vi "WHD_VEten_0.2.vi"() -> ()   [LabVIEW 2015]
uses:
  <vilib>/RTwatchdog.llb/Watchdog expiration actions.ctl
  <vilib>/LabVIEW Targets/FPGA/cRIO/shared/nicrio_ModuleControls/nicrio_cRIO-9234_DataRatesRing2.ctl
  <vilib>/userdefined/High Color/nirio_resource_hc.ctl
  <vilib>/FPGAPlugInAG/cRIO-9031/niLvFpga_Open_cRIO-9031.vi
  <vilib>/Utility/file.llb/Write Delimited Spreadsheet (string).vi
  <vilib>/real-time/rtutility.llb/RT Restart Target (Self).vi
  <vilib>/FPGAPlugInAG/cRIO-9031/niLvFpga_Run_cRIO-9031.vi
  <vilib>/Utility/error.llb/Error Cluster From Error Code.vi
  <vilib>/rvi/errors/niLvFpgaAdjustHostInterfaceError.vi
  <vilib>/rvi/interface/common/niFpgaWaitOnOcc.vi
  <vilib>/FPGAPlugInAG/cRIO-9031/niLvFpga_Reset_cRIO-9031.vi
  <vilib>/Utility/file.llb/Read Delimited Spreadsheet (string).vi
  <vilib>/FPGAPlugInAG/cRIO-9031/niLvFpga_Close_cRIO-9031.vi
  <vilib>/rvi/interface/nirviOpenFPGA/nirviOpenFPGA.xnode
  FPGA Bitfiles/W&RDEuskotrenIBA_FPGATarget2_FPGA8aws_YNPuKjtl2tk.lvbitx
  <vilib>/rvi/interface/nirviMethod/nirviMethod.xnode
  <vilib>/rvi/interface/nirviReadWriteControl/nirviReadWriteControl.xnode
  <vilib>/rvi/interface/nirviCloseFPGA/nirviCloseFPGA.xnode
  <vilib>/real-time/NI_Real-Time Libraries.lvlib
  <vilib>/NI_Real-Time Target Support.lvlib
  NiFpgaLv.dll
  <vilib>/rvi/errors/niLvFpgaMergeErrorWithErrorCode.vi
  AURA_Wheel/Json2Labv.lvlib
  AURA_Wheel/AuraWheelAPI/AuraWheel.lvlib
  <vilib>/FPGAPlugInAG/cRIO-9031/niLvFpga_ConfigureFifo_cRIO-9031.vi
  <vilib>/FPGAPlugInAG/cRIO-9031/niLvFpga_StartFifo_cRIO-9031.vi
  <vilib>/FPGAPlugInAG/cRIO-9031/niLvFpga_ReadFifo_cRIO-9031.vi
  <vilib>/FPGAPlugInAG/cRIO-9031/niLvFpga_StopFifo_cRIO-9031.vi
panel:
  out "error out":errorcluster
  in  "TIEMPO SUBIDA FALLOS (MS)":u16=13
  out "all rows":string[][](array[string])
  out "Response headers 2":string
  in  "Parametros AuraWheel 2":string[](array[string])=["JOH653JDBHGGA4111LOMJG", "WRD03NEM", "http://api.aurawheel.sb/services/wrd/upload"]
  out "data 2":cluster{"status":string}
  out "JSON String Out 2":string
  in  "DC CONTROL":bool
  out "JSON String Out":string
  out "WHEEL_SENSOR":bool=TRUE
  out "Series del convoy":string[](array[string])
  out "it-read-LR6":i32[](array[numeric])
  out "it-LR6":i32
  out "Ejes_convoy":i32
  out "Nº Ejes":i32[](array[numeric])
  out "Plataformas?":bool
  out "TAGs LR6":string[](array[string])
  out "Series_flota":string[](array[string])
  out "Tabla_flota":string[][](array[string])
  out "Puntos medios de las ventanas":dbl[][](array[numeric])
  out "configuration file path":path=path "c:/Parametros.cfg"
  in  "IP synchr":string
  in  "Canal ccero?":bool
  in  "Digital?":bool=TRUE
  out "Numeric 3":i32
  out "TAGs HEX":string[](array[string])
  out "data":cluster{"status":string}
  out "confRFID":path=path "c:/RFID/TAGS.csv"
  out "TAGS leidos":path=path "c:/RFID/TAGS.csv"
  in  "Use Aura?":bool
  in  "Parametros AuraWheel":string[](array[string])
  in  "Parámetros acelerómetros":dbl[](array[numeric])
  out "RFID_Error 2":errorcluster
  out "Acelerómetros OK?":bool[](array[boolean])
  out "Fin":bool
  out "Contador":i32=1
  in  "expiration actions":T1={"reset"=TRUE, "occurrence"=FALSE, "trigger protocol"=enum."active high", "trigger line"=enum."none", "disable watchdog on VI exit"=FALSE}
  out "Path TEST":path=path "c:/TEST"
  out "Fallo fotocelula":bool
  out "Path_Borrar":path=path "c:/Trenes"
  out "Longitud de la unidad":dbl
  out "Bucle Espera":i32
  out "Aviso no detección":string
  out "Time to Acquire Block (ms)":i32
  out "Distancia de acelerómetros":dbl[](array[numeric])
  out "Block Size":u32
  out "Distancias generales":dbl[](array[numeric])
  in  "Reset del controlador":bool
  in  "Configuración":bool
  in  "Parar la aplicación":bool
  out "Acel 4":bool=TRUE
  out "Acel 3":bool=TRUE
  out "Acel 2":bool=TRUE
  out "Acel 1":bool=TRUE
  out "RFID":bool=TRUE
  out "date/time string":string
  out "Obstruido?":bool
  out "Tiempo":dbl
  out "Inicio pasada":timestamp
  out "Ultimo TEST":timestamp
  out "Fuente":bool=TRUE
  out "Estado":string
  in  "Number of Channels":u32=9
  out "RFID_ID":refnum<k5>
  out "DC OK":string
  out "Aviso temperatura":string
  in  "Tab Control":T2(tab)=enum."Parámetros"
  out "UT":dbl
  out "V (m/s)":dbl
  out "Temperatura (ºC)":dbl
  out "Max RMS Ruedas":dbl[][](array[numeric])
  in  "Hora de borrado":string
  out "result":bool
  out "TAGs":string[](array[string])
  out "TAGs_AURAwheel":string[][](array[string])
  out "Nombre de archivo":path[](array[path])
  out "Tiempo de paso (s)":dbl
  out "Tiempo extra de adquisición (s)":dbl
  out "Número de ejes detectados":i32
  out "Buffer Underflow":bool
  out "Buffer Overflow":bool
  out "Disco Duro Disponible (bytes)":i64
  out "Path Pasada":path
  out "Fallo sensores":string
  out "T fuera rango":bool
  in  "Frecuencia de muestreo (Hz)":dbl=25600.0
  in  "Escaneos de la FIFO por canal":u32=4000
  in  "Tiempo extra al detector de paso (s)":dbl=1.0
  in  "Filtro digital (ms)":u16=13
  in  "dt RMS":dbl=256.0
  in  "Frecuencia de muestreo y módulo CRIO":T3=2 items=["51.200 kS/s (NI 9234)"=1, "25.600 kS/s (NI 9234)"=2, "17.067 kS/s (NI 9234)"=3, "12.800 kS/s (NI 9234)"=4, "10.240 kS/s (NI 9234)"=5, "8.533 kS/s (NI 9234)"=6, "7.314 kS/s (NI 9234)"=7, "6.400 kS/s (NI 9234)"=8, "5.689 kS/s (NI 9234)"=9, "5.120 kS/s (NI 9234)"=10, "4.654 kS/s (NI 9234)"=11, "4.267 kS/s (NI 9234)"=12, "3.938 kS/s (NI 9234)"=13, "3.657 kS/s (NI 9234)"=14, "3.413 kS/s (NI 9234)"=15, "3.200 kS/s (NI 9234)"=16, "3.012 kS/s (NI 9234)"=17, "2.845 kS/s (NI 9234)"=18, "2.695 kS/s (NI 9234)"=19, "2.560 kS/s (NI 9234)"=20, "2.438 kS/s (NI 9234)"=21, "2.328 kS/s (NI 9234)"=22, "2.226 kS/s (NI 9234)"=23, "2.133 kS/s (NI 9234)"=24, "2.048 kS/s (NI 9234)"=25, "1.969 kS/s (NI 9234)"=26, "1.896 kS/s (NI 9234)"=27, "1.829 kS/s (NI 9234)"=28, "1.765 kS/s (NI 9234)"=29, "1.707 kS/s (NI 9234)"=30, "1.652 kS/s (NI 9234)"=31]
  in  "Puerto RFID":u16=2189
  in  "IP RFID":string="192.168.106.99"
  in  "Offset_rueda":fxp<+/-,24,-4>=0.004999998956918716 format="%.27g"
  in  "Count(mSec)":u32=2
  in  "LR6 IP address":string="192.168.106.94"
  in  "Port LR6":u16=2001
  in  "LIMITE MAX":dbl
  in  "LIMITE MIN":dbl
  in  "TIMEOUT":u16=2189
  in  "BYTES TO READ":u16=2189
  in  "DEVICE ADDRESS":u16=2189
  in  "Nº ACELEROMETROS":u16=13
  in  "Nº INDUCTIVOS":u16=13
  in  "Nº MAX ARCHIVOS":u16=13
  in  "MB MIN MEMORIA LIBRE":dbl=13.0 format="%#_10g"
  in  "MB LIBRE OK":dbl=13.0 format="%#_10g"
  in  "RFID_NEM_On":bool
  in  "RFID_GEN_On":bool
  in  "WDOG RESET":bool
  in  "WDOG DISABLE":bool
  out "ID DISPOSITIVO":string
  in  "HORA_SUBIDA_FALLOS":string="08:51 AM"
  out "time string 3":string
  in  "HORA_FINAL_SUBIDA":string="08:51 AM"
  in  "Pruebas RFID 2":bool
  in  "Pruebas RFID 1":bool
  in  "Descargar":bool
  out "Parámetros":bool=TRUE
  out "Distacias y medidas de dispositivos":bool=TRUE
  out "RFID_Error":errorcluster
  out "error FPGA":errorcluster
  out "error manipulacion archivos":errorcluster
  out "Unidades y ejes":bool=TRUE
  out "RFID":bool=TRUE
  out "error AURA":errorcluster
  out "Response headers":string
  out "RFID_LR6_Error":errorcluster
  # "Funciona?"
  # "Inductivo"
  # "A4"
  # "A3"
  # "A1"
  # "A2"
  # "Última detección de unidad"
  # "Error!!"
  # "Estado de la memoria"
  # "Espera"
  # "Adquisicion"
  # "Adquisicion"
  # "Procesado"
  # "Procesado"
  # "Procesado"
  # "Procesado"
  # "Procesado"
  # "Parámetros de configuración"
  # "Límites Acelerómetros"
  # "Parámetros de muestreo"
  # "Parámetros de adquisición"
  # "Parámetros de procesado"
  # "Descarga de planos y TEST"
  # "NO"
  # "SI"
  # "Descarga archivos binarios de adquisición"
  # "NO"
  # "SI"
  # "Cargar datos de configuración"
  # "Errores!!"
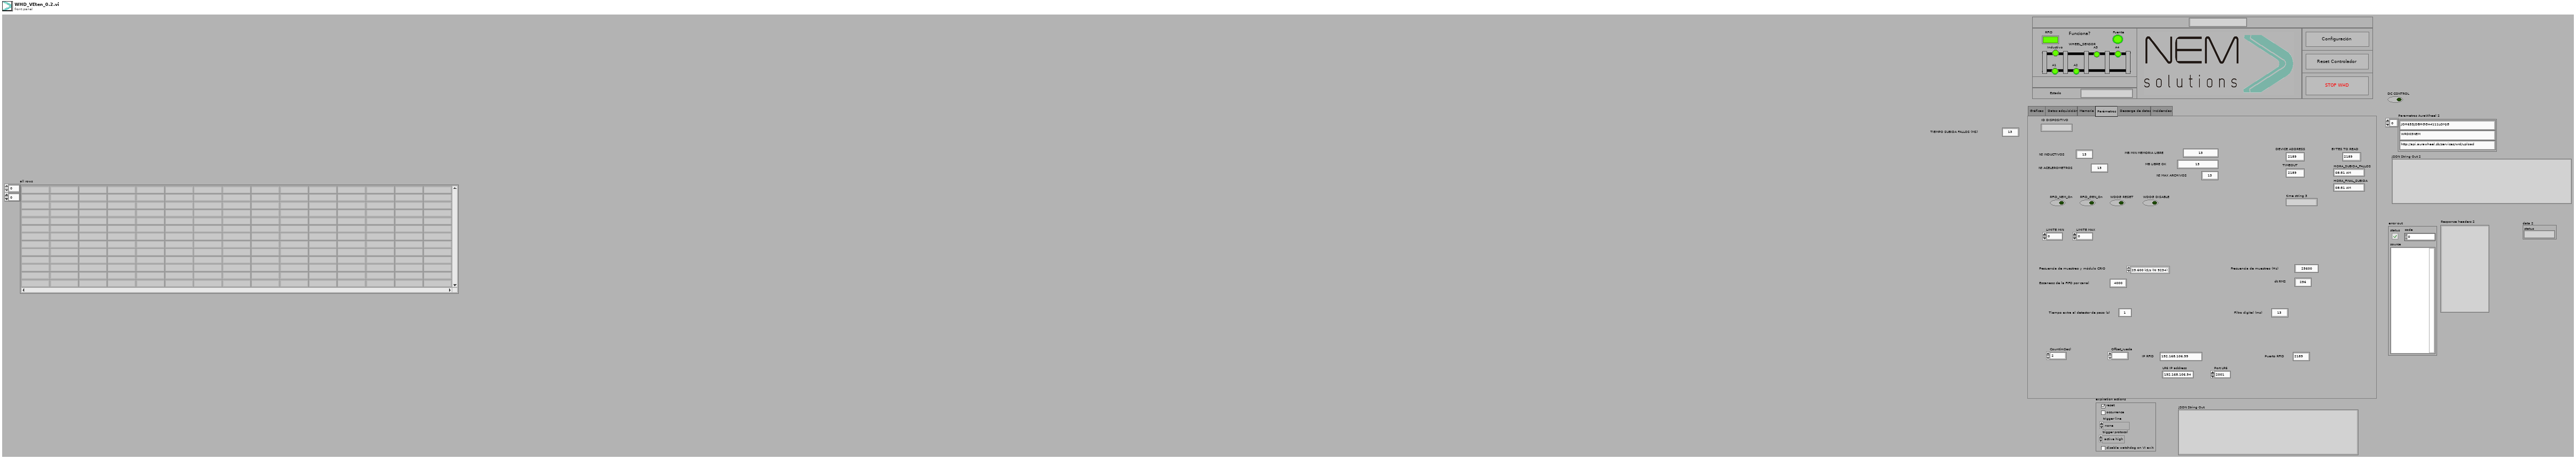
[diagram p1: front panel]
types:
  T1 = typedef "Watchdog expiration actions.ctl" = cluster{"reset":bool, "occurrence":bool, "trigger protocol":enum16{"active high", "active low", "open collector"}, "trigger line":enum16{"none", "line 0", "line 1", "line 2", "line 3", "line 4", "line 5", "line 6", "line 7", "SMB line 0"}, "disable watchdog on VI exit":bool}
  T2 = enum32{"Gráficas", "Datos adquisición", "Memoria", "Parámetros", "Descarga de datos", "Incidencias"}
  T3 = typedef "nicrio_cRIO-9234_DataRatesRing2.ctl" = u8
  T4 = typedef "nirio_resource_hc.ctl" = tag
  T5 = enum16{"Standard", "Buffered", "CRLF", "Immediate"}
  T6 = enum16{"open", "replace", "create", "open or create", "replace or create", "replace or create with confirmation"}
  T7 = enum16{"big-endian, network order", "native, host order", "little-endian"}
  T8 = cluster{"error IO":errorcluster, bool[], u32[], string[], dbl[]}
  T9 = cluster{"g_ts":dbl, "p_sp":dbl, "p_tp":dbl, "p_tg":cluster{"tg_n":dbl, "tg_t":string}[], "p_ax":cluster{"ax_n":dbl, "ax_sp":dbl, "ax_wh":cluster{"wh_p":dbl, "wh_a1":dbl, "wh_a2":dbl, "wh_a3":dbl, "wh_a4":dbl}[]}[]}
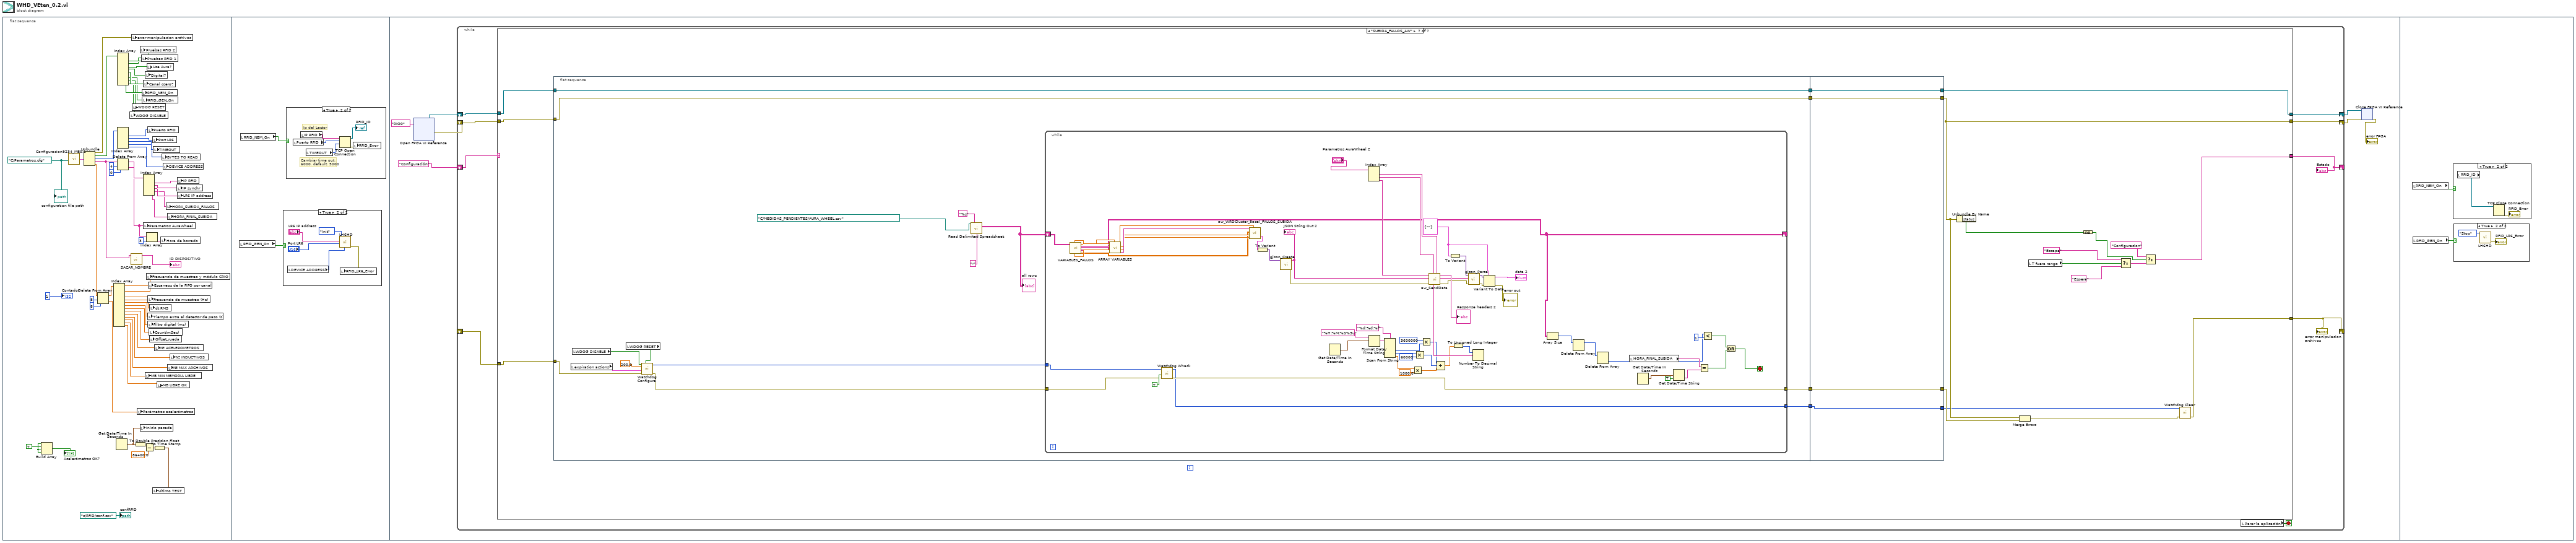
[diagram p0: block diagram]
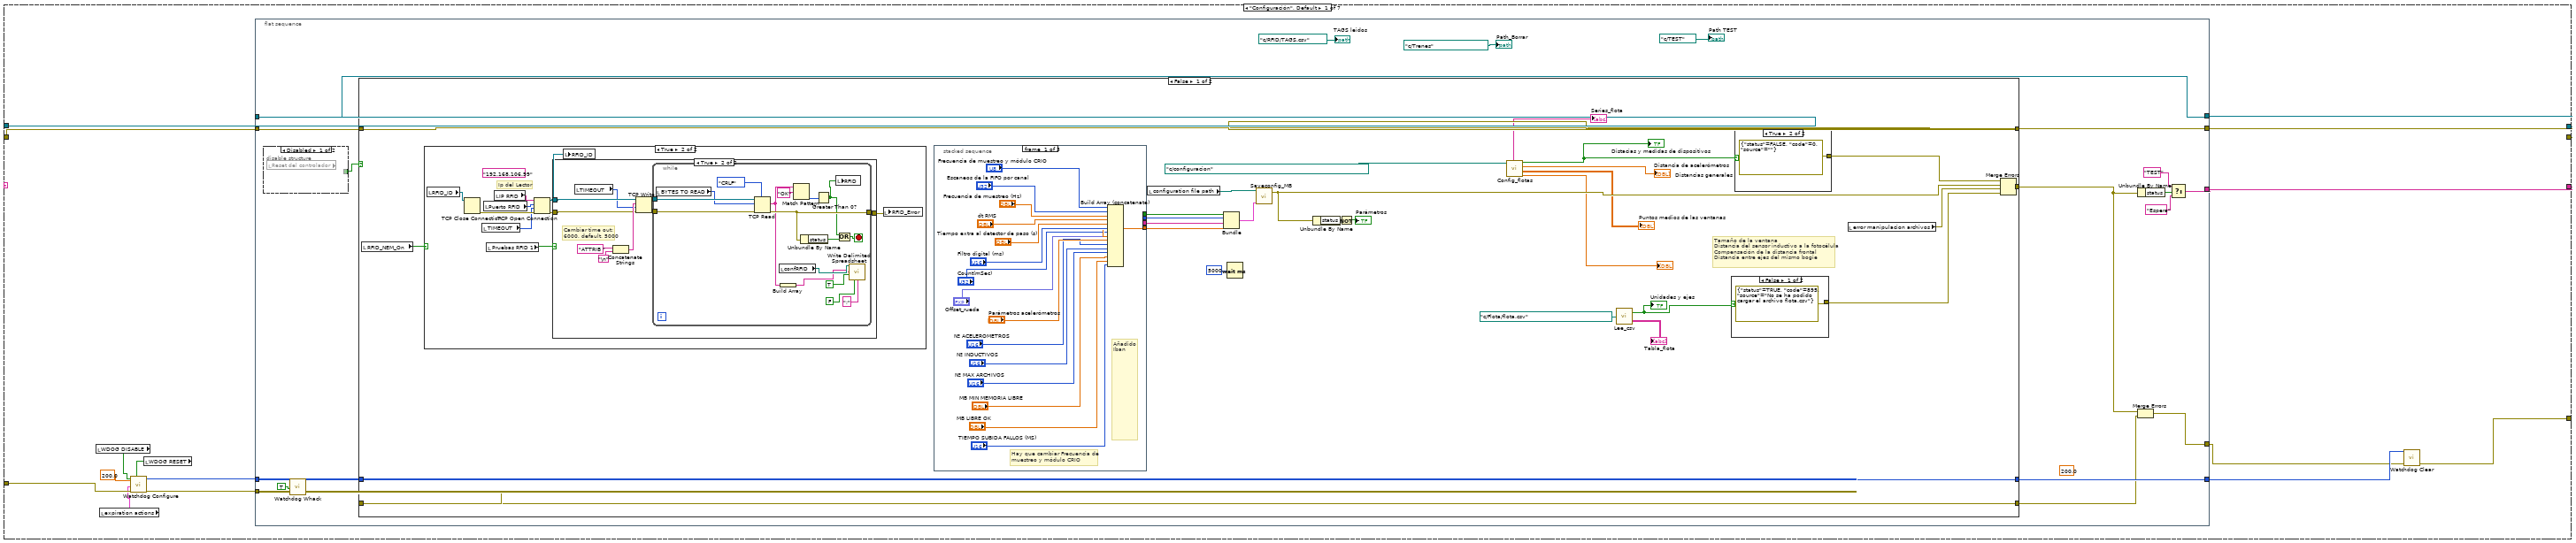
[diagram p4: hidden frame]
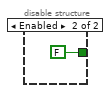
[diagram p5: hidden frame]
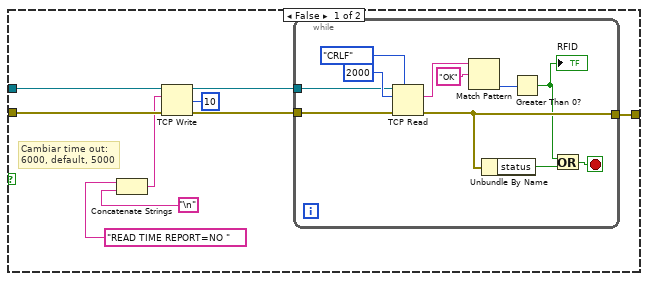
[diagram p7: hidden frame]
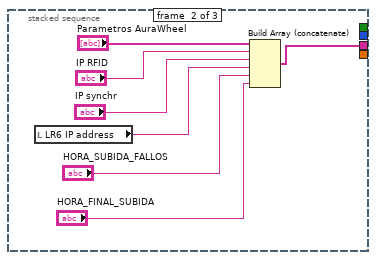
[diagram p8: hidden frame]
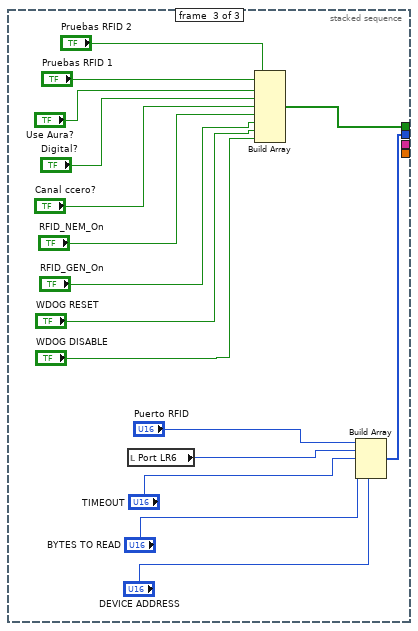
[diagram p9: hidden frame]
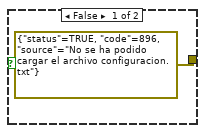
[diagram p10: hidden frame]
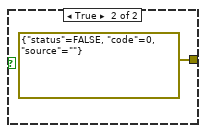
[diagram p11: hidden frame]
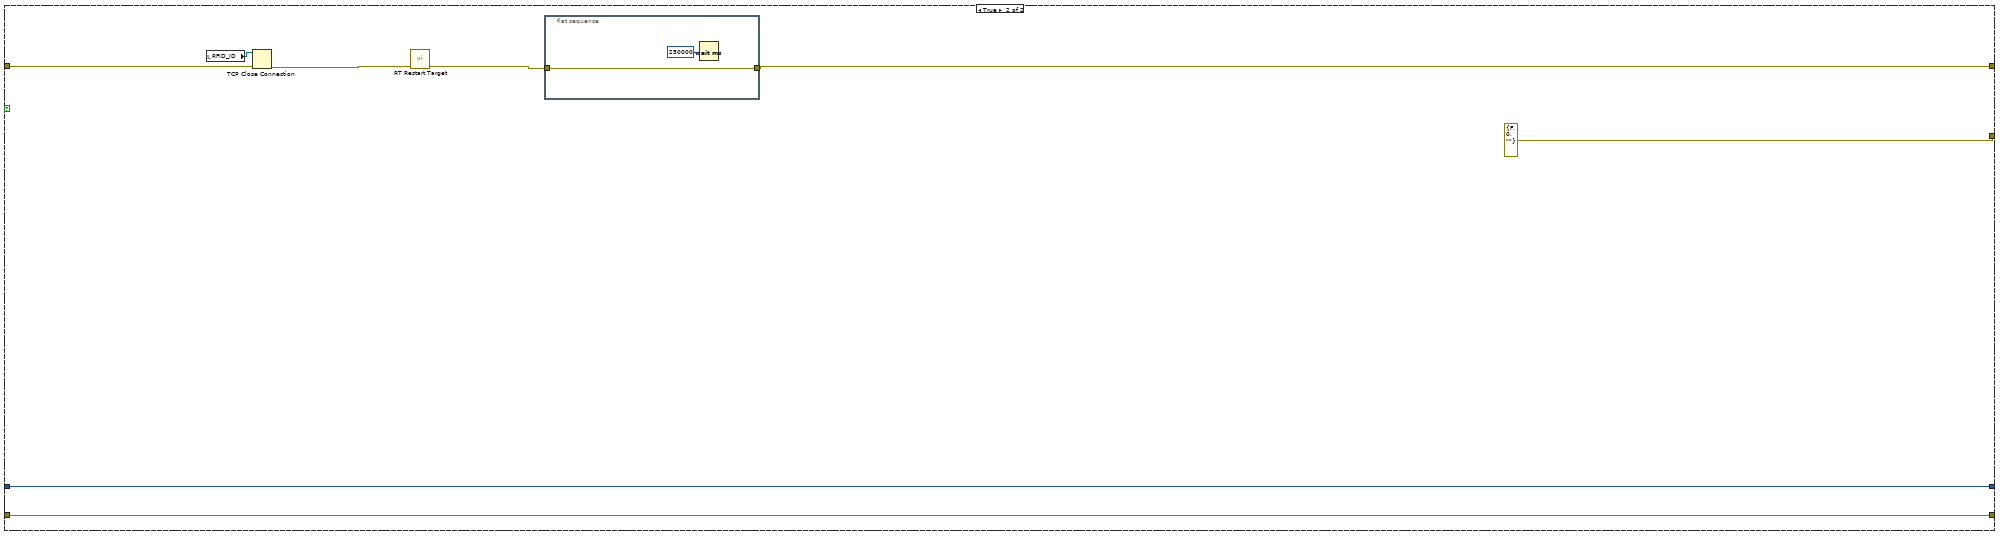
[diagram p12: hidden frame]
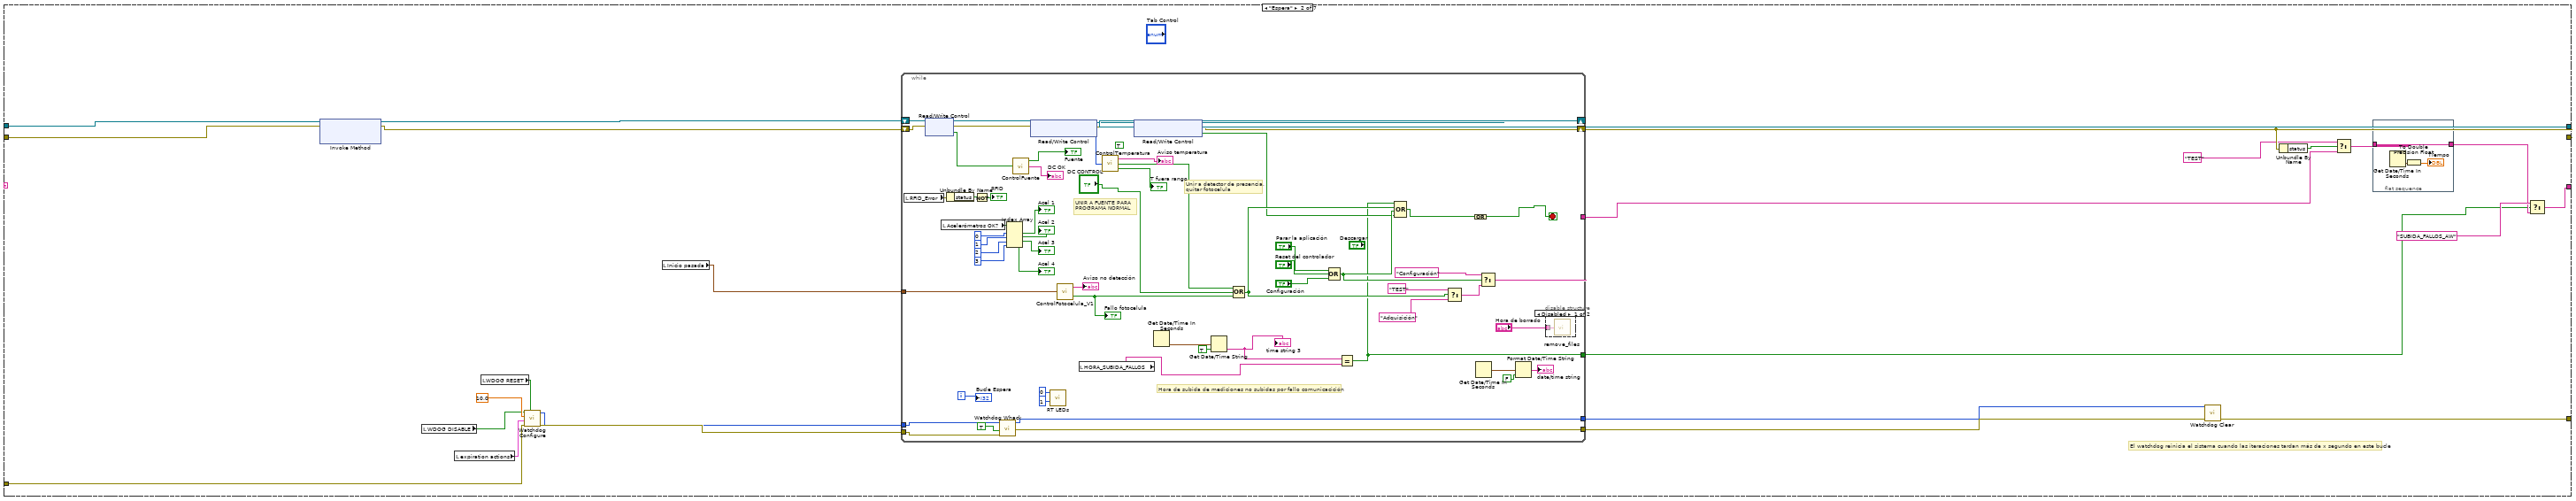
[diagram p13: hidden frame]
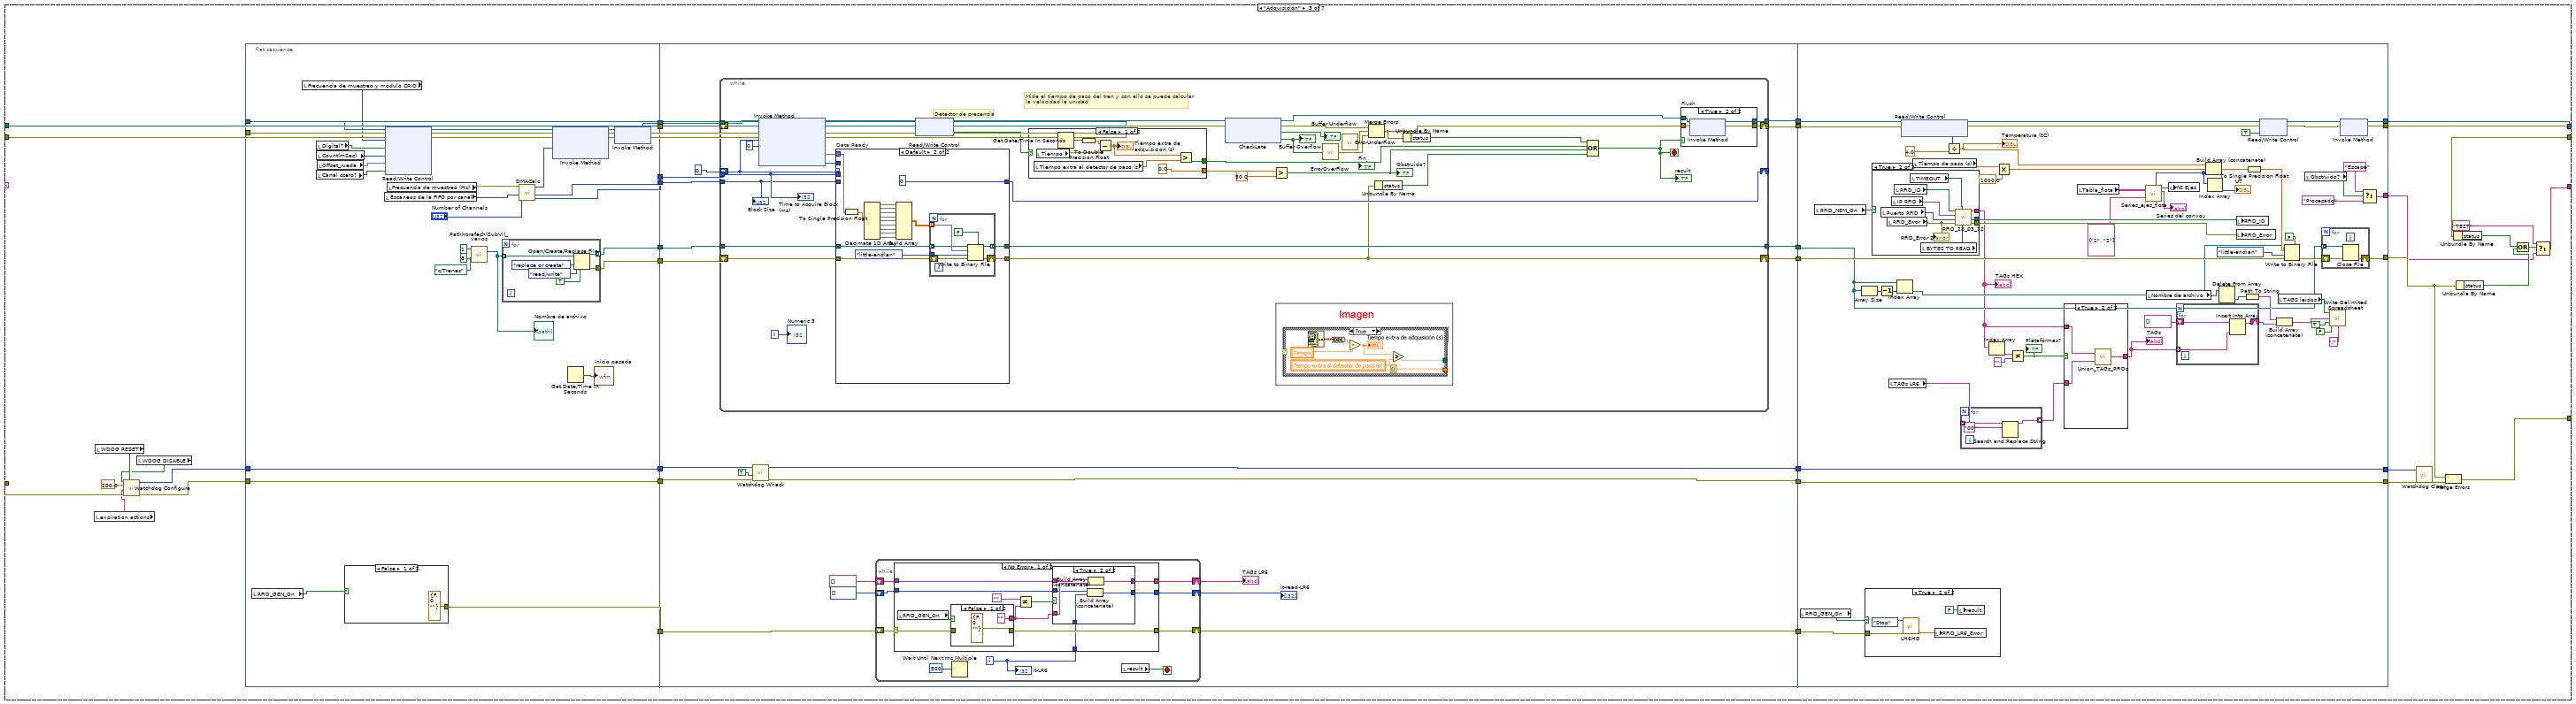
[diagram p15: hidden frame]
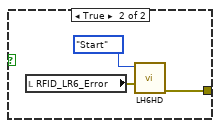
[diagram p16: hidden frame]
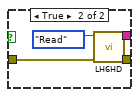
[diagram p17: hidden frame]
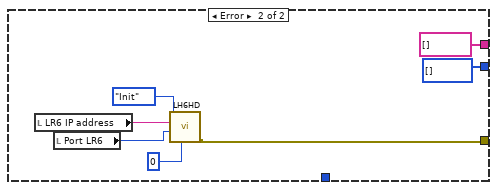
[diagram p19: hidden frame]
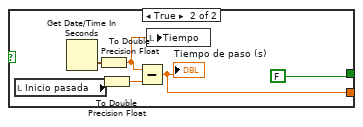
[diagram p20: hidden frame]
diagram:
  n1 = flat-sequence {
    frame #0 {
      w43 = TRUE
      w17 = path "C:/Parametros.cfg" ("configuration file path")
      n2 = Build Array(w43, w43, w43, w43) -> (→"Acelerómetros OK?":bool[])
      n3 = call "Configuracion9234_MB0.1.vi"("configuration file path"=w17) -> ("output cluster"=w40:T8)
      n4 = Unbundle(w40) -> ("error IO"=w46:errorcluster, w45:bool[], w44:u32[], w16:string[], w38:dbl[])
      n5 = Delete From Array(array=w38, length=8, index=8) -> (deleted portion=w34:dbl[], array with subset deleted=w37:dbl[])
      n6 = Index Array(array=w37) -> (element #1=w54:dbl, element #2=w53:dbl, element #3=w52:dbl, element #4=w51:dbl, element #5=w50:dbl, element #6=w49:dbl, element #7=w25:dbl, element #8=w24:dbl, element #9=w7:dbl, element #10=w6:dbl, element #11=w5:dbl, element #12=w4:dbl, element #13=w3:dbl)  [unwired: 13 in]
      n7 = Get Date/Time In Seconds() -> (seconds since 1Jan1904=w56:timestamp)
      n8 = Index Array(array=w45) -> (element #1=w48:bool, element #2=w47:bool, element #3=w33:bool, element #4=w21:bool, element #5=w26:bool, element #6=w11:bool, element #7=w10:bool, element #8=w9:bool, element #9=w8:bool)  [unwired: 9 in]
      n9 = Index Array(array=w44) -> (element #1=w39:u32, element #2=w18:u32, element #3=w14:u32, element #4=w13:u32, element #5=w12:u32)  [unwired: 5 in]
      n10 = Delete From Array(array=w16, length=4, index=0) -> (deleted portion=w22:string[], array with subset deleted=w32:string[])
      n11 = local write "WDOG DISABLE"(w8) -> ()
      n12 = call "SACAR_NOMBRE.vi"("Array 2"=w16) -> ("deleted portion"=→"ID DISPOSITIVO":string)  [unwired: 9 in]
      n13 = local write "error manipulacion archivos"(w46) -> ()
      n14 = local write "WDOG RESET"(w9) -> ()
      n15 = To Double Precision Float(number=w56) -> (double precision float=w58:dbl)
      n16 = local write "Parámetros acelerómetros"(w34) -> ()
      n17 = local write "Pruebas RFID 2"(w48) -> ()
      n18 = local write "Inicio pasada"(w56) -> ()
      n19 = local write "Pruebas RFID 1"(w47) -> ()
      n20 = local write "RFID_NEM_On"(w11) -> ()
      n21 = local write "RFID_GEN_On"(w10) -> ()
      n22 = local write "Canal ccero?"(w26) -> ()
      n23 = Index Array(array=w32) -> (element #1=w20:string, element #2=w23:string, element #3=w19:string, element #4=w2:string, element #5=w1:string)  [unwired: 5 in]
      n24 = local write "Parametros AuraWheel"(w22) -> ()
      n25 = Subtract(x=w58, y=86400.0) -> (x-y=w57:dbl)
      n26 = local write "Digital?"(w21) -> ()
      n27 = local write "MB MIN MEMORIA LIBRE"(w4) -> ()
      n28 = Index Array(array=w22, index=3) -> (element=w27:string)
      n29 = local write "Frecuencia de muestreo y módulo CRIO"(w54) -> ()
      n30 = local write "Use Aura?"(w33) -> ()
      n31 = local write "Tiempo extra al detector de paso (s)"(w50) -> ()
      n32 = local write "Puerto RFID"(w39) -> ()
      n33 = local write "Frecuencia de muestreo (Hz)"(w52) -> ()
      n34 = local write "Filtro digital (ms)"(w49) -> ()
      n35 = local write "Escaneos de la FIFO por canal"(w53) -> ()
      n36 = local write "Count(mSec)"(w25) -> ()
      n37 = local write "dt RMS"(w51) -> ()
      n38 = local write "Offset_rueda"(w24) -> ()
      n39 = local write "Port LR6"(w18) -> ()
      n40 = local write "TIMEOUT"(w14) -> ()
      n41 = To Time Stamp(1:w57) -> (0:w55:timestamp)
      n42 = local write "Ultimo TEST"(w55) -> ()
      n43 = local write "Nº ACELEROMETROS"(w7) -> ()
      n44 = local write "MB LIBRE OK"(w3) -> ()
      n45 = local write "Hora de borrado"(w27) -> ()
      n46 = local write "BYTES TO READ"(w13) -> ()
      n47 = local write "DEVICE ADDRESS"(w12) -> ()
      n48 = local write "HORA_SUBIDA_FALLOS"(w2) -> ()
      n49 = local write "HORA_FINAL_SUBIDA"(w1) -> ()
      n50 = local write "Nº MAX ARCHIVOS"(w5) -> ()
      n51 = local write "Nº INDUCTIVOS"(w6) -> ()
      n52 = local write "IP synchr"(w23) -> ()
      n53 = local write "IP RFID"(w20) -> ()
      n54 = local write "LR6 IP address"(w19) -> ()
      "Contador" <- 1
      "confRFID" <- path "c:/RFID/conf.csv" ("file path (use dialog)")
      "configuration file path" <- w17
    }
    frame #1 {
      n55 = local read "RFID_GEN_On"() -> (w60:bool)
      n56 = local read "RFID_NEM_On"() -> (w61:bool)
      n57 = case shown="True" w60 {
        frame False {
        }
        frame True {
          n58 = local read "DEVICE ADDRESS"() -> (w66:u16)
          n59 = call "LH6HD.vi"("DeviceAddress"=w66, "Reader Port"="Port LR6", "IP Address"="LR6 IP address", "Action"=enum16{"Init", "Start", "Read", "Stop", "Exit"}."Init") -> ("error out"=w64:errorcluster)  [unwired: 6 in, 1 out]
          n60 = local write "RFID_LR6_Error"(w64) -> ()
        }
      }
      n61 = case shown="True" w61 {
        frame False {
        }
        frame True {
          # "Cambiar time out:\n6000, default, 5000"
          # "Ip del Lector"
          n62 = local read "Puerto RFID"() -> (w69:u16)
          n63 = local read "IP RFID"() -> (w70:string)
          n64 = local read "TIMEOUT"() -> (w67:u16)
          n65 = TCP Open Connection(address=w70, remote port or service name=w69, timeout ms (60000)=w67) -> (connection ID=→"RFID_ID":refnum<k5>, error out=w68:errorcluster)  [unwired: 1 in, 1 out]
          n66 = local write "RFID_Error"(w68) -> ()
        }
      }
    }
    frame #2 {
      n67 = xnode "Open FPGA VI Reference"("resource name"=T4 "RIO0") -> ("FPGA VI Reference Out"=w78:refnum<k20>, "error out"=w77:errorcluster)  [unwired: 1 in]
      n68 = while {
        shift-right: [w82] -> _
        shift-left: "Configuración" -> [w87]
        shift-right: [w80] -> w74
        shift-left: w78 -> [w86]
        shift-right: [w79] -> w73
        shift-left: w77 -> [w85]
        shift-right: [w84] -> _
        shift-left: _ -> [w83]
        stop <- w81 stop-if-true
        n69 = case shown="\"SUBIDA_FALLOS_AW\"" w87 {
          tunnel: [w93 w261 w354 w679 w905 "TEST" ("t") w1008] -> w82
          tunnel: [w102 w276 w375 w694 w904 w972 w1006] -> w80
          tunnel: [w101 w275 w376 w669 w903 w969 w994] -> w79
          tunnel: w86 -> [w92 w280 w385 w694 w904 w971 w1005]
          tunnel: w85 -> [w91 w278 w384 w669 w894 w968 w1007]
          tunnel: [w95 w269 w371 w676 w881 w973 w990] -> w84
          tunnel: w83 -> [w100 w274 w377 w692 w895 w973 w998]
          frame "Configuración", Default {
            (unwired) 200.0 ("timeout (1 sec)")
            n70 = local read "WDOG DISABLE"() -> (w89:bool)
            n71 = local read "expiration actions"() -> (w94:T1)
            n72 = local read "WDOG RESET"() -> (w90:bool)
            n73 = call <vilib>:"Watchdog Configure.vi"("RESET"=w90, "error in (no error)"=w100, "expiration actions"=w94, "timeout (1 sec)"=200.0, "DISABLE WDOG"=w89) -> ("error out"=w98:errorcluster, "watchdogID"=w99:u64)  [unwired: 1 in, 2 out]
            n74 = flat-sequence {
              tunnel: [w113] -> w101
              tunnel: [w121] -> w93
              tunnel: w92 -> [w114]
              tunnel: [w114] -> w102
              tunnel: [w116] -> w96
              tunnel: w99 -> [w110]
              tunnel: w98 -> [w109]
              tunnel: [w107] -> w97
              tunnel: w91 -> [w103]
              frame #0 {
                n75 = disable-structure shown="Disabled" {
                  disable-tunnel: [_ FALSE] -> w111
                  frame Disabled {
                    n76 = local read "Reset del controlador"() -> ()  [unwired: 1 out]
                  }
                  frame Enabled {
                  }
                }
                n77 = call <vilib>:"Watchdog Whack.vi"("error in (no error)"=w109, "reset watchdog after expire? (F)"=TRUE, "watchdogID in"=w110) -> ("error out"=w106:errorcluster, "watchdogID out"=w108:u64)  [unwired: 3 out]
                n78 = case shown="False" w111 {
                  tunnel: w103 -> [w150 w253]
                  tunnel: [w150 w250] -> w113
                  tunnel: [w136 errorcluster {"status"=FALSE, "code"=0, "source"=""} ("error IO")] -> w112
                  tunnel: w108 -> [w127 w248]
                  tunnel: [w127 w248] -> w107
                  tunnel: [w126 w249] -> w105
                  tunnel: w106 -> [w126 w249]
                  frame False {
                    # "Tamaño de la ventana\nDistancia del sensor inductivo a la fotocélula\nCompensación de la distancia frontal\nDistancia entre ejes del mismo bogie"
                    n79 = local read "RFID_NEM_On"() -> (w124:bool)
                    n80 = case shown="True" w124 {
                      frame False {
                      }
                      frame True {
                        (unwired) "192.168.106.99" ("address")
                        # "Ip del Lector"
                        n81 = local read "RFID_ID"() -> (w158:refnum<k5>)
                        n82 = TCP Close Connection(connection ID=w158) -> (error out=w159:errorcluster)  [unwired: 2 in, 1 out]
                        n83 = local read "TIMEOUT"() -> (w151:u16)
                        n84 = local read "Puerto RFID"() -> (w156:u16)
                        n85 = local read "Pruebas RFID 1"() -> (w152:bool)
                        n86 = local read "IP RFID"() -> (w155:string)
                        n87 = TCP Open Connection(address=w155, remote port or service name=w156, timeout ms (60000)=w151, error in (no error)=w159) -> (connection ID=w157:refnum<k5>, error out=w153:errorcluster)  [unwired: 1 out]
                        n88 = case shown="True" w152 {
                          tunnel: w157 -> [w168 w183]
                          tunnel: [w166 w181] -> w154
                          tunnel: w153 -> [w163 w182]
                          frame False {
                            # "Cambiar time out:\n6000, default, 5000"
                            n89 = Concatenate Strings("READ TIME REPORT=NO " ("data in"), "\n") -> (w160:string)
                            n90 = TCP Write(connection ID=w168, data in=w160, error in (no error)=w163, 9:10 ("timeout ms (25000)")) -> (connection ID out=w164:refnum<k5>, error out=w165:errorcluster)  [unwired: 1 out]
                            n91 = while {
                              tunnel: w165 -> [w177]
                              tunnel: w164 -> [w176]
                              tunnel: [w175] -> w166
                              stop <- w172 stop-if-true
                              n92 = TCP Read(connection ID=w176, bytes to read=2000, error in (no error)=w177, 7:T5."CRLF" ("mode (standard)")) -> (data out=w170:string, error out=w175:errorcluster)  [unwired: 1 in, 1 out]
                              n93 = Match Pattern(string=w170, regular expression="OK") -> (offset past match=w173:i32)  [unwired: 4 out]
                              n94 = Unbundle By Name(w175) -> ("status"=w171:bool)
                              n95 = Greater Than 0?(x=w173) -> (x > 0?=w169:bool)
                              "RFID" <- w169
                              n96 = Or(x=w169, y=w171) -> (x .or. y?=w172:bool)
                            }
                          }
                          frame True {
                            # "Cambiar time out:\n6000, default, 5000"
                            n97 = local read "TIMEOUT"() -> (w180:u16)
                            n98 = Concatenate Strings("ATTRIB " ("data in"), "\n") -> (w188:string)
                            n99 = TCP Write(connection ID=w183, data in=w188, error in (no error)=w182, 9:w180) -> (connection ID out=w185:refnum<k5>, error out=w184:errorcluster)  [unwired: 1 out]
                            n100 = while {
                              tunnel: w184 -> [w203]
                              tunnel: w185 -> [w202]
                              tunnel: [w201] -> w181
                              stop <- w198 stop-if-true
                              n101 = local read "BYTES TO READ"() -> (w189:u16)
                              n102 = TCP Read(connection ID=w202, bytes to read=w189, error in (no error)=w203, 7:T5."CRLF" ("mode (standard)")) -> (data out=w195:string, error out=w201:errorcluster)  [unwired: 1 in, 1 out]
                              n103 = local read "confRFID"() -> (w194:path)
                              n104 = Build Array(w195) -> (w190:string[])
                              n105 = Match Pattern(string=w195, regular expression="OK") -> (offset past match=w199:i32)  [unwired: 4 out]
                              n106 = Unbundle By Name(w201) -> ("status"=w197:bool)
                              n107 = Greater Than 0?(x=w199) -> (x > 0?=w196:bool)
                              n108 = local write "RFID"(w196) -> ()
                              n109 = Or(x=w196, y=w197) -> (x .or. y?=w198:bool)
                              n110 = call-poly <vilib>:"Write Delimited Spreadsheet.vi"("file path (dialog if empty)"=w194, "1D data"=w190, "append to file? (F)"=TRUE ("append to file? (new file:F)"), "transpose? (F)"=FALSE ("transpose? (no:F)"), "delimiter (\\t)"=";" ("delimiter (\\t)")) -> ()  [unwired: 9 in, 2 out]
                            }
                          }
                        }
                        n111 = local write "RFID_ID"(w157) -> ()
                        n112 = local write "RFID_Error"(w154) -> ()
                      }
                    }
                    n113 = stacked-sequence {
                      tunnel: [w215 _ _] -> w140
                      tunnel: [_ w227 _] -> w139
                      tunnel: [_ _ w240] -> w141
                      tunnel: [_ _ w239] -> w142
                      frame #0 {
                        # "Añadido\nIban"
                        # "Hay que cambiar Frecuencia de\nmuestreo y módulo CRIO"
                        n114 = Build Array (concatenate)("Frecuencia de muestreo y módulo CRIO", "Escaneos de la FIFO por canal", "Frecuencia de muestreo (Hz)", "dt RMS", "Tiempo extra al detector de paso (s)", "Filtro digital (ms)", "Count(mSec)", "Offset_rueda", "Parámetros acelerómetros", "Nº ACELEROMETROS", "Nº INDUCTIVOS", "Nº MAX ARCHIVOS", "MB MIN MEMORIA LIBRE", "MB LIBRE OK", "TIEMPO SUBIDA FALLOS (MS)") -> (w215:dbl[])
                      }
                      frame #1 {
                        n115 = local read "LR6 IP address"() -> (w223:string)
                        n116 = Build Array (concatenate)("Parametros AuraWheel", "IP RFID", "IP synchr", w223, "HORA_SUBIDA_FALLOS", "HORA_FINAL_SUBIDA") -> (w227:string[])
                      }
                      frame #2 {
                        n117 = local read "Port LR6"() -> (w235:u16)
                        n118 = Build Array("Pruebas RFID 2", "Pruebas RFID 1", "Use Aura?", "Digital?", "Canal ccero?", "RFID_NEM_On", "RFID_GEN_On", "WDOG RESET", "WDOG DISABLE") -> (w239:bool[])
                        n119 = Build Array("Puerto RFID", w235, "TIMEOUT", "BYTES TO READ", "DEVICE ADDRESS") -> (w240:u16[])
                      }
                    }
                    n120 = local read "configuration file path"() -> (w137:path)
                    n121 = Bundle(w142, w141, w139, w140) -> (w138:cluster{bool[], u16[], string[], dbl[]})  [unwired: 1 in]
                    n122 = Wait (ms)(milliseconds to wait=u32 5000) -> ()  [unwired: 1 out]
                    n123 = call "Saveconfig_MB.vi"("configuration file path"=w137, "Configuracion"=w138) -> ("error out"=w145:errorcluster)  [unwired: 4 in]
                    n124 = Unbundle By Name(w145) -> ("status"=w146:bool)
                    n125 = Not(x=w146) -> (.not. x?=→"Parámetros":bool)
                    n126 = call "Config_flotas.vi"("file path (dialog if empty)"=path "c:/configuracion") -> ("Distancias generales"=→"Distancias generales":dbl[], "Puntos medios de las ventanas"=→"Puntos medios de las ventanas":dbl[][], "Distancia de acelerómetros"=→"Distancia de acelerómetros":dbl[], "Distacias y medidas de dispositivos"=w135:bool, "Series_flota"=→"Series_flota":string[])  [unwired: 3 in]
                    "Distacias y medidas de dispositivos" <- w135
                    n127 = call "Lee_csv.vi"("Path"=path "c:/Flota/flota.csv") -> ("Tabla_flota"=→"Tabla_flota":string[][], "Lectura_OK?"=w131:bool)
                    "Unidades y ejes" <- w131
                    n128 = case shown="False" w131 {
                      tunnel: [errorcluster {"status"=TRUE, "code"=895, "source"="No se ha podido cargar el archivo flota.csv"} ("error out") errorcluster {"status"=FALSE, "code"=0, "source"=""} ("error out")] -> w143
                      frame False {
                      }
                      frame True {
                      }
                    }
                    n129 = case shown="True" w135 {
                      tunnel: [errorcluster {"status"=TRUE, "code"=896, "source"="No se ha podido cargar el archivo configuracion.txt"} ("error out") errorcluster {"status"=FALSE, "code"=0, "source"=""} ("error out")] -> w148
                      frame False {
                      }
                      frame True {
                      }
                    }
                    n130 = local read "error manipulacion archivos"() -> (w144:errorcluster)
                    n131 = Merge Errors(w148, w145, w144, w143) -> (w136:errorcluster)
                  }
                  frame True {
                    n132 = local read "RFID_ID"() -> (w255:refnum<k5>)
                    n133 = TCP Close Connection(connection ID=w255, error in (no error)=w253) -> (error out=w252:errorcluster)  [unwired: 2 out]
                    n134 = call-poly <vilib>:"RT Restart Target.vi"("error in (no error)"=w252) -> ("error out"=w251:errorcluster)  [unwired: 10 in]
                    n135 = flat-sequence {
                      tunnel: [w257] -> w250
                      tunnel: w251 -> [w257]
                      frame #0 {
                        n136 = Wait (ms)(milliseconds to wait=u32 250000) -> ()  [unwired: 1 out]
                      }
                    }
                  }
                }
                n137 = Unbundle By Name(w112) -> ("status"=w122:bool)
                n138 = Merge Errors(w112, w105) -> (w116:errorcluster)
                n139 = Select(t="TEST", s=w122, f="Espera") -> (s? t:f=w121:string)
                "Path_Borrar" <- path "c:/Trenes" ("file path (use dialog)")
                "Path TEST" <- path "c:/TEST" ("file path (use dialog)")
                "TAGS leidos" <- path "c:/RFID/TAGS.csv" ("file path (use dialog)")
              }
            }
            n140 = call <vilib>:"Watchdog Clear.vi"("error in (no error)"=w96, "watchdogID in"=w97) -> ("error out"=w95:errorcluster)  [unwired: 5 out]
          }
          frame "Espera" {
            # "El watchdog reinicia el sistema cuando las iteraciones tardan más de x segundo en este bucle"
            n141 = xnode "Invoke Method"("FPGA VI Reference In"=w280, "error in"=w278) -> ("FPGA VI Reference Out"=w279:refnum<k20>, "error out"=w277:errorcluster)  [unwired: 1 in]
            n142 = local read "WDOG DISABLE"() -> (w265:bool)
            n143 = local read "expiration actions"() -> (w267:T1)
            n144 = local read "WDOG RESET"() -> (w266:bool)
            n145 = call <vilib>:"Watchdog Configure.vi"("RESET"=w266, "error in (no error)"=w274, "expiration actions"=w267, "timeout (1 sec)"=10.0, "DISABLE WDOG"=w265) -> ("error out"=w273:errorcluster, "watchdogID"=w272:u64)  [unwired: 1 in, 2 out]
            n146 = local read "Inicio pasada"() -> (w282:timestamp)
            n147 = while {
              tunnel: [w314] -> w281
              shift-right: [w307] -> w276
              shift-left: w279 -> [w299]
              shift-right: [w306] -> w275
              shift-left: w277 -> [w297]
              tunnel: w282 -> [w320]
              tunnel: w273 -> [w304]
              tunnel: w272 -> [w303]
              tunnel: [w302] -> w271
              tunnel: [w301] -> w270
              tunnel: [w286] -> w258
              i -> [w340]
              stop <- w288 stop-if-true
              (unwired) TRUE
              # "Hora de subida de mediciones no subidas por fallo comunicacición"
              # "UNIR A FUENTE PARA\nPROGRAMA NORMAL"
              # "Unir a detector de presencia,\nquitar fotocelula"
              n148 = local read "RFID_Error"() -> (w327:errorcluster)
              n149 = xnode "Read/Write Control"("FPGA VI Reference In"=w299, "error in"=w297) -> ("FPGA VI Reference Out"=w298:refnum<k20>, "error out"=w296:errorcluster, "DC OK"=w295:bool)
              n150 = local read "Acelerómetros OK?"() -> (w319:bool[])
              n151 = Unbundle By Name(w327) -> ("status"=w325:bool)
              n152 = Not(x=w325) -> (.not. x?=→"RFID":bool)
              n153 = call <vilib>:"Watchdog Whack.vi"("error in (no error)"=w304, "reset watchdog after expire? (F)"=TRUE, "watchdogID in"=w303) -> ("error out"=w302:errorcluster, "watchdogID out"=w301:u64)  [unwired: 2 in, 1 out]
              n154 = Index Array(array=w319, index #1=0 ("index"), index #2=1 ("index"), index #3=2 ("index"), index #4=3 ("index")) -> (element #1=→"Acel 1":bool, element #2=→"Acel 2":bool, element #3=→"Acel 3":bool, element #4=→"Acel 4":bool)
              n155 = call "ControlFuente.vi"("DC OK 3"=w295) -> ("DC OK 2"=→"Fuente":bool, "DC OK"=→"DC OK":string)  [unwired: 1 out]
              n156 = xnode "Read/Write Control"("FPGA VI Reference In"=w298, "error in"=w296) -> ("FPGA VI Reference Out"=w333:refnum<k20>, "error out"=w332:errorcluster, "Chassis Temperature"=w338:i16)
              n157 = call <vilib>:"RT LEDs.vi"("State"=1, "LED Num"=0) -> ()  [unwired: 1 in, 5 out]
              n158 = call "ControlFotocelula_V1.vi"("Tiempo de entrada a espera"=w320) -> ("Aviso no detección"=→"Aviso no detección":string, "Boolean"=w330:bool)
              "Fallo fotocelula" <- w330
              n159 = local read "HORA_SUBIDA_FALLOS"() -> (w290:string)
              n160 = call "ControlTemperatura.vi"("Chassis Temperature"=w338) -> ("Aviso temperatura"=→"Aviso temperatura":string, "Boolean"=w334:bool, "T fuera rango"=→"T fuera rango":bool)
              n161 = xnode "Read/Write Control"("FPGA VI Reference In"=w333, "error in"=w332) -> ("FPGA VI Reference Out"=w307:refnum<k20>, "error out"=w306:errorcluster, "Detector de presencia"=w305:bool)
              n162 = Get Date/Time In Seconds() -> (seconds since 1Jan1904=w292:timestamp)
              n163 = Get Date/Time String(seconds (now)=w292, want seconds? (F)=TRUE) -> (time string=w291:string)  [unwired: 1 in, 1 out]
              "time string 3" <- w291
              n164 = Compound Arithmetic op=OR(w334, "DC CONTROL", w330) -> (w331:bool)
              n165 = Compound Arithmetic op=OR("Parar la aplicación", "Reset del controlador", "Configuración") -> (w328:bool)
              n166 = Equal?(x=w291, y=w290) -> (x = y?=w286:bool)
              n167 = Compound Arithmetic op=OR(w286, w331, w328, w305) -> (w289:bool)
              n168 = Select(t="TEST", s=w331, f="Adquisición") -> (s? t:f=w343:string)
              n169 = Compound Arithmetic op=OR(w289) -> (w288:bool)
              n170 = Get Date/Time In Seconds() -> (seconds since 1Jan1904=w311:timestamp)
              n171 = Select(t="Configuración", s=w328, f=w343) -> (s? t:f=w314:string)
              n172 = Format Date/Time String(seconds (now)=w311, UTC format=FALSE) -> (date/time string=→"date/time string":string)  [unwired: 1 in]
              n173 = disable-structure shown="Disabled" {
                disable-tunnel: "Hora de borrado" -> [w347 _]
                frame Disabled {
                  n174 = call "remove_files.vi"("Hora de borrado"=w347) -> ()  [unwired: 1 in]
                }
                frame Enabled {
                }
              }
              "Bucle Espera" <- w340
            }
            n175 = call <vilib>:"Watchdog Clear.vi"("error in (no error)"=w271, "watchdogID in"=w270) -> ("error out"=w269:errorcluster)  [unwired: 5 in]
            n176 = Unbundle By Name(w275) -> ("status"=w264:bool)
            n177 = Select(t="TEST", s=w264, f=w281) -> (s? t:f=w262:string)
            n178 = flat-sequence {
              tunnel: [w284] -> w259
              tunnel: w262 -> [w284]
              frame #0 {
                n179 = Get Date/Time In Seconds() -> (seconds since 1Jan1904=w285:timestamp)
                n180 = To Double Precision Float(number=w285) -> (double precision float=→"Tiempo":dbl)
              }
            }
            n181 = Select(t="SUBIDA_FALLOS_AW", s=w258, f=w259) -> (s? t:f=w261:string)
          }
          frame "Adquisición" {
            n182 = local read "expiration actions"() -> (w353:T1)
            n183 = local read "WDOG RESET"() -> (w350:bool)
            n184 = local read "WDOG DISABLE"() -> (w349:bool)
            n185 = call <vilib>:"Watchdog Configure.vi"("RESET"=w350, "error in (no error)"=w377, "expiration actions"=w353, "timeout (1 sec)"=200.0, "DISABLE WDOG"=w349) -> ("error out"=w361:errorcluster, "watchdogID"=w362:u64)  [unwired: 1 in, 2 out]
            n186 = flat-sequence {
              tunnel: w361 -> [w414]
              tunnel: w362 -> [w415]
              tunnel: w384 -> [w409]
              tunnel: w385 -> [w410]
              tunnel: [w415] -> w370
              tunnel: [w414] -> w369
              tunnel: [w408] -> w368
              tunnel: [w407] -> w367
              tunnel: [w406] -> w366
              tunnel: [w405] -> w365
              tunnel: [w404] -> w364
              tunnel: [w387] -> w363
              tunnel: [w388] -> w352
              tunnel: [w446] -> w383
              tunnel: [w432] -> w382
              tunnel: [w445] -> w381
              tunnel: [w444] -> w380
              tunnel: [w441] -> w379
              tunnel: [w434] -> w378
              tunnel: w370 -> [w443]
              tunnel: w369 -> [w442]
              tunnel: w368 -> [w440]
              tunnel: w367 -> [w439]
              tunnel: w366 -> [w438]
              tunnel: w365 -> [w437]
              tunnel: w364 -> [w436]
              tunnel: w363 -> [w435]
              tunnel: w352 -> [w431]
              tunnel: [w430] -> w351
              tunnel: w383 -> [w626]
              tunnel: w382 -> [w625]
              tunnel: w381 -> [w612]
              tunnel: w380 -> [w611]
              tunnel: w379 -> [w600]
              tunnel: [w630] -> w357
              tunnel: w378 -> [w632]
              tunnel: [w617] -> w372
              tunnel: [w618] -> w376
              tunnel: [w619] -> w375
              tunnel: [w626] -> w374
              tunnel: [w625] -> w373
              tunnel: w351 -> [w597]
              frame #0 {
                n187 = local read "RFID_GEN_On"() -> (w386:bool)
                n188 = local read "Frecuencia de muestreo y módulo CRIO"() -> (w396:T3)
                n189 = local read "Digital?"() -> (w389:bool)
                n190 = local read "Count(mSec)"() -> (w392:u32)
                n191 = local read "Canal ccero?"() -> (w390:bool)
                n192 = local read "Offset_rueda"() -> (w391:fxp<+/-,24,-4>)
                n193 = case shown="False" w386 {
                  tunnel: [errorcluster {"status"=FALSE, "code"=0, "source"=""} ("error out") w419] -> w388
                  frame False {
                  }
                  frame True {
                    n194 = local read "RFID_LR6_Error"() -> (w417:errorcluster)
                    n195 = call "LH6HD.vi"("error in (no error)"=w417, "Action"=enum16{"Init", "Start", "Read", "Stop", "Exit"}."Start") -> ("error out"=w419:errorcluster)  [unwired: 8 in, 1 out]
                  }
                }
                n196 = local read "Escaneos de la FIFO por canal"() -> (w394:u32)
                n197 = xnode "Read/Write Control"("FPGA VI Reference In"=w410, "error in"=w409, "Data Rate"=w396, "Digital?"=w389, "Count(mSec)"=w392, "Offset_rueda"=w391, "Canal ccero?"=w390) -> ("FPGA VI Reference Out"=w401:refnum<k20>, "error out"=w400:errorcluster)
                n198 = local read "Frecuencia de muestreo (Hz)"() -> (w402:dbl)
                n199 = call "Pathhorafech(SubVI)_varios.vi"("Folder path"=path "c:/Trenes", "Nº de acelerómetros"=8, "Nº inductivos"=1) -> ("Acel_Paths"=w397:path[])  [unwired: 1 in, 1 out]
                "Nombre de archivo" <- w397
                n200 = for {
                  tunnel: w397 -> [w422] mode=indexing
                  tunnel: [w421] -> w404 mode=indexing
                  tunnel: [w420] -> w387
                  n201 = Open/Create/Replace File(file path (use dialog)=w422, operation (0:open)=T6."replace or create", access (0:read/write)=enum16{"read/write", "read-only", "write-only"}."read/write", disable buffering (F)=TRUE) -> (refnum out=w421:refnum<file>, error out=w420:errorcluster)  [unwired: 1 in, 2 out]
                }
                n202 = call "DMACalc.vi"("Number of Channels"="Number of Channels", "Number of Samples"=w394, "Rate (Hz)"=w402) -> ("Block Size"=w405:u32, "Time to Acquire Block (ms)"=w406:i32, "Host Buffer Size"=w411:u32)  [unwired: 6 in]
                n203 = xnode "Invoke Method"("FPGA VI Reference In"=w401, "error in"=w400, "Requested Depth"=w411) -> ("FPGA VI Reference Out"=w413:refnum<k20>, "error out"=w412:errorcluster)  [unwired: 1 out]
                n204 = Get Date/Time In Seconds() -> (seconds since 1Jan1904=→"Inicio pasada":timestamp)
                n205 = xnode "Invoke Method"("FPGA VI Reference In"=w413, "error in"=w412) -> ("FPGA VI Reference Out"=w408:refnum<k20>, "error out"=w407:errorcluster)
              }
              frame #1 {
                n206 = while "Data Acquisition" {
                  tunnel: w440 -> [w493]
                  shift-right: [w521] -> _
                  shift-left: u32 0 ("t") -> [w517]
                  tunnel: w438 -> [w522]
                  tunnel: w437 -> [w520]
                  shift-right: [w523] -> w444
                  shift-left: w439 -> [w514]
                  tunnel: [w518] -> w445
                  tunnel: w436 -> [w498]
                  tunnel: [w499] -> w441
                  shift-right: [w497] -> w434
                  shift-left: w435 -> [w510]
                  i -> [w492]
                  stop <- w519 stop-if-true
                  # "Detector de presencia"
                  # "Mide el tiempo de paso del tren y con ello se puede calcular\nla velocidad la unidad"
                  n207 = xnode "Invoke Method"("FPGA VI Reference In"=w493, "error in"=w514, "Number of Elements"=w517, "Timeout (ms)"=0) -> ("FPGA VI Reference Out"=w489:refnum<k20>, "error out"=w496:errorcluster, "Data"=w513:fxp<+/-,24,4>[], "Elements Remaining"=w515:u32)
                  n208 = case "Data Ready" shown="Default" w517 {
                    tunnel: w522 -> [w541 _]
                    tunnel: [w540 u32 0 ("t")] -> w521
                    tunnel: w520 -> [w542 _]
                    tunnel: w515 -> [w539 _]
                    tunnel: w513 -> [_ w563]
                    tunnel: w510 -> [w538 w562]
                    tunnel: [w538 w564] -> w497
                    tunnel: w498 -> [w537 w561]
                    tunnel: [w537 w560] -> w499
                    frame 0 {
                      # "En este caso se compara los elementos que quedan\nen la FIFO del controlador con el tamaño dell bloque\nque aparece en el panel frontal. Si el número de \nelementos en la FIFO es mayor o igual que el tamaño\n del bloque se pasa al siguiente caso y se guardan \nlos datos en un archivo. El reloj que aparece es una\nespera para no consumir recursos."
                      n209 = Greater Or Equal?(x=w539, y=w542) -> (x >= y?=w543:bool)
                      n210 = case shown="True" w543 {
                        tunnel: [u32 0 ("Block Size") w547] -> w540
                        tunnel: [w546 0 ("t")] -> w544
                        tunnel: w541 -> [w546 _]
                        tunnel: w542 -> [_ w547]
                        frame False {
                        }
                        frame True {
                        }
                      }
                      n211 = call "WaitMinTimeBetweenCall.vi"("Minimum ms between calls"=w544) -> ()  [unwired: 2 in]
                    }
                    frame Default {
                      n212 = To Single Precision Float(number=w563) -> (single precision float=w550:sgl[])
                      n213 = Decimate 1D Array(w550) -> (w556:sgl[], w559:sgl[], w558:sgl[], w557:sgl[], w555:sgl[], w554:sgl[], w553:sgl[], w552:sgl[], w551:sgl[])
                      n214 = Build Array(w556, w559, w558, w557, w555, w554, w553, w552, w551) -> (w549:sgl[][])
                      n215 = for {
                        tunnel: T7."little-endian" ("byte order (0:big-endian, network order)") -> [w573]
                        shift-right: [w567] -> w564
                        shift-left: w562 -> [w568]
                        tunnel: w549 -> [w571] mode=indexing
                        tunnel: w561 -> [w570] mode=indexing
                        tunnel: [w569] -> w560 mode=indexing
                        n216 = Write to Binary File(file (use dialog)=w570, data=w571, error in=w568, 5:FALSE ("prepend array or string size? (T)"), 9:w573) -> (refnum out=w569:refnum<file>, error out=w567:errorcluster)  [unwired: 2 out]
                      }
                    }
                  }
                  n217 = xnode "Read/Write Control"("FPGA VI Reference In"=w489, "error in"=w496) -> ("FPGA VI Reference Out"=w512:refnum<k20>, "error out"=w511:errorcluster, "Fotocelula"=w504:bool)
                  n218 = case shown="False" w504 {
                    tunnel: [w526 FALSE] -> w503
                    tunnel: [0.0 w532] -> w502
                    frame False {
                      n219 = local read "Tiempo extra al detector de paso (s)"() -> (w525:dbl)
                      n220 = local read "Tiempo"() -> (w530:dbl)
                      n221 = Get Date/Time In Seconds() -> (seconds since 1Jan1904=w527:timestamp)
                      n222 = To Double Precision Float(number=w527) -> (double precision float=w528:dbl)
                      n223 = Subtract(x=w528, y=w530) -> (x-y=w529:dbl)
                      "Tiempo extra de adquisición (s)" <- w529
                      n224 = Greater?(x=w529, y=w525) -> (0:w526:bool)
                    }
                    frame True {
                      n225 = local read "Inicio pasada"() -> (w535:timestamp)
                      n226 = Get Date/Time In Seconds() -> (seconds since 1Jan1904=w534:timestamp)
                      n227 = To Double Precision Float(number=w534) -> (double precision float=w531:dbl)
                      n228 = To Double Precision Float(number=w535) -> (double precision float=w536:dbl)
                      n229 = Subtract(x=w531, y=w536) -> (x-y=w532:dbl)
                      "Tiempo de paso (s)" <- w532
                      n230 = local write "Tiempo"(w531) -> ()
                    }
                  }
                  "Fin" <- w503
                  n231 = xnode ("CheckLate")("FPGA VI Reference In"=w512, "error in"=w511) -> ("FPGA VI Reference Out"=w491:refnum<k20>, "error out"=w507:errorcluster, "Buffer Underflow"=→"Buffer Underflow":bool, "Buffer Overflow"=w494:bool)
                  "Buffer Overflow" <- w494
                  n232 = Greater?(x=w502, y=50.0) -> (0:w500:bool)
                  "Obstruido?" <- w500
                  n233 = call "ErrorOverFlow.vi"("Buffer Overflow"=w494) -> ("error out"=w505:errorcluster)
                  n234 = call "ErrorUnderFlow.vi"() -> ("error out"=w506:errorcluster)  [unwired: 1 in]
                  n235 = Merge Errors(w507, w506, w505) -> (w490:errorcluster)
                  n236 = Unbundle By Name(w497) -> ("status"=w501:bool)
                  n237 = Unbundle By Name(w490) -> ("status"=w509:bool)
                  n238 = Compound Arithmetic op=OR(w509, w503, w500, w501) -> (w519:bool)
                  "result" <- w519
                  n239 = case "Flush" shown="True" w519 {
                    tunnel: [w574 w579] -> w523
                    tunnel: [w575 w578] -> w518
                    tunnel: w491 -> [w575 w577]
                    tunnel: w490 -> [w574 w576]
                    frame False {
                    }
                    frame True {
                      n240 = xnode "Invoke Method"("FPGA VI Reference In"=w577, "error in"=w576) -> ("FPGA VI Reference Out"=w578:refnum<k20>, "error out"=w579:errorcluster)
                    }
                  }
                  "Block Size" <- w520
                  "Time to Acquire Block (ms)" <- w522
                  "Numeric 3" <- w492
                }
                n241 = call <vilib>:"Watchdog Whack.vi"("error in (no error)"=w442, "reset watchdog after expire? (F)"=TRUE, "watchdogID in"=w443) -> ("error out"=w432:errorcluster, "watchdogID out"=w446:u64)  [unwired: 3 out]
                n242 = while {
                  shift-right: [w454] -> w430
                  shift-left: w431 -> [w455]
                  shift-right: [w453] -> w428
                  shift-left: string[] [] -> [w452]
                  shift-right: [w449] -> w426
                  shift-left: i32[] [] -> [w451]
                  i -> [w450]
                  stop <- w448 stop-if-true
                  n243 = case shown="No Error" w455 {
                    selector: w455 -> [w467 _]
                    tunnel: [w466 w486] -> w454
                    tunnel: [w462 string[] []] -> w453
                    tunnel: w452 -> [w461 _]
                    tunnel: w451 -> [w460 _]
                    tunnel: w450 -> [w459 _]
                    tunnel: [w458 i32[] []] -> w449
                    frame No Error {
                      n244 = local read "RFID_GEN_On"() -> (w457:bool)
                      n245 = case shown="False" w457 {
                        tunnel: w467 -> [_ w472]
                        tunnel: [errorcluster {"status"=FALSE, "code"=0, "source"=""} ("error out") w471] -> w466
                        tunnel: ["" ("Tag") w470] -> w463
                        frame False {
                        }
                        frame True {
                          n246 = call "LH6HD.vi"("error in (no error)"=w472, "Action"=enum16{"Init", "Start", "Read", "Stop", "Exit"}."Read") -> ("error out"=w471:errorcluster, "Tag"=w470:string)  [unwired: 8 in]
                        }
                      }
                      n247 = Not Equal?(x="", y=w463) -> (x != y?=w464:bool)
                      n248 = case shown="True" w464 {
                        tunnel: w463 -> [_ w481]
                        tunnel: [w475 w480] -> w462
                        tunnel: w461 -> [w475 w479]
                        tunnel: w460 -> [w474 w478]
                        tunnel: w459 -> [_ w477]
                        tunnel: [w474 w476] -> w458
                        frame False {
                        }
                        frame True {
                          n249 = Build Array (concatenate)(w478, w477) -> (w476:i32[])
                          n250 = Build Array (concatenate)(w479, w481) -> (w480:string[])
                        }
                      }
                    }
                    frame Error {
                      n251 = local read "LR6 IP address"() -> (w484:string)
                      n252 = local read "Port LR6"() -> (w483:u16)
                      n253 = call "LH6HD.vi"("DeviceAddress"=u8 0, "Reader Port"=w483, "IP Address"=w484, "Action"=enum16{"Init", "Start", "Read", "Stop", "Exit"}."Init") -> ("error out"=w486:errorcluster)  [unwired: 6 in, 1 out]
                    }
                  }
                  n254 = Wait Until Next ms Multiple(millisecond multiple=u32 500) -> ()  [unwired: 1 out]
                  n255 = local read "result"() -> (w448:bool)
                  "it-LR6" <- w450
                }
                "TAGs LR6" <- w428
                "it-read-LR6" <- w426
              }
              frame #2 {
                n256 = local read "RFID_GEN_On"() -> (w580:bool)
                n257 = local read "RFID_NEM_On"() -> (w581:bool)
                n258 = Array Size(array=w600) -> (size(s)=w598:i32)
                n259 = case shown="True" w580 {
                  tunnel: w597 -> [_ w643]
                  frame False {
                  }
                  frame True {
                    n260 = call "LH6HD.vi"("error in (no error)"=w643, "Action"=enum16{"Init", "Start", "Read", "Stop", "Exit"}."Stop") -> ("error out"=w640:errorcluster)  [unwired: 8 in, 1 out]
                    n261 = local write "RFID_LR6_Error"(w640) -> ()
                    n262 = local write "result"(FALSE ("result")) -> ()
                  }
                }
                n263 = case shown="True" w581 {
                  tunnel: [refnum<k5> refnum ("connection ID out") w653] -> w627
                  tunnel: [errorcluster {"status"=FALSE, "code"=0, "source"=""} ("RFID Error") w652] -> w620
                  tunnel: [string[] [] ("TAGs HEX") w649] -> w594
                  frame False {
                  }
                  frame True {
                    n264 = local read "Puerto RFID"() -> (w651:u16)
                    n265 = local read "RFID_Error"() -> (w655:errorcluster)
                    "RFID_Error 2" <- w655
                    n266 = local read "IP RFID"() -> (w650:string)
                    n267 = local read "RFID_ID"() -> (w654:refnum<k5>)
                    n268 = local read "TIMEOUT"() -> (w648:u16)
                    n269 = local read "BYTES TO READ"() -> (w647:u16)
                    n270 = call "RFID_28_03_12.vi"("BYTES TO READ"=w647, "TIMEOUT"=w648, "RFID_Error"=w655, "Puerto RFID"=w651, "IP RFID"=w650, "RFID ID"=w654) -> ("RFID Error"=w652:errorcluster, "connection ID out"=w653:refnum<k5>, "TAGs HEX"=w649:string[])  [unwired: 1 in, 1 out]
                  }
                }
                "TAGs HEX" <- w594
                n271 = Decrement(x=w598) -> (x-1=w599:i32)
                n272 = local read "TAGs LR6"() -> (w585:string[])
                n273 = Index Array(array=w600, index=w599) -> (element=w608:refnum<file>)
                n274 = xnode "Read/Write Control"("FPGA VI Reference In"=w612, "error in"=w611) -> ("FPGA VI Reference Out"=w629:refnum<k20>, "error out"=w628:errorcluster, "Chassis Temperature"=w638:i16)
                n275 = local read "Tiempo de paso (s)"() -> (w623:dbl)
                n276 = Divide(x=w638, y=4.0) -> (x/y=w639:dbl)
                "Temperatura (ºC)" <- w639
                n277 = for {
                  tunnel: w585 -> [w658] mode=indexing
                  tunnel: [w656] -> w584 mode=indexing
                  n278 = Search and Replace String(input string=w658, search string="00") -> (result string=w656:string)  [unwired: 6 in, 3 out]
                }
                n279 = Index Array(array=w594) -> (element=w596:string)  [unwired: 1 in]
                n280 = Multiply(x=w623, y=1000.0) -> (x*y=w621:dbl)
                n281 = Not Equal?(x=w596, y="" ("delimiter (\\t)")) -> (x != y?=w593:bool)
                "Plataformas?" <- w593
                n282 = case shown="True" w593 {
                  tunnel: w584 -> [w659 w660]
                  tunnel: [w659 w662] -> w588
                  tunnel: w594 -> [_ w661]
                  frame False {
                  }
                  frame True {
                    n283 = call "Union_TAGs_RFIDs.vi"("TAGs LR6"=w660, "TAGs HEX"=w661) -> ("TAGs"=w662:string[])
                  }
                }
                "TAGs" <- w588
                n284 = local read "Tabla_flota"() -> (w591:string[][])
                n285 = call "Series_ejes_flota.vi"("Tabla_flota"=w591, "Tags"=string[] ["1", "2"]) -> ("Nº Ejes"=w590:i32[], "Series del convoy"=→"Series del convoy":string[], "UT"=w587:i32[])  [unwired: 2 in]
                n286 = local read "Nombre de archivo"() -> (w607:path[])
                n287 = local write "Nº Ejes"(w590) -> ()
                n288 = for {
                  shift-right: [w668] -> w615
                  shift-left: string[] [] -> [w667]
                  tunnel: w588 -> [w666] mode=indexing
                  n289 = Insert Into Array(array=w667, new element=w666) -> (w668:string[])  [unwired: 1 in]
                }
                n290 = Build Array (concatenate)(w639, w621, w587) -> (w633:dbl[])
                n291 = Index Array(array=w587) -> (element=→"UT":i32)  [unwired: 1 in]
                n292 = Delete From Array(array=w607) -> (deleted portion=w606:path)  [unwired: 2 in, 1 out]
                n293 = local write "RFID_ID"(w627) -> ()
                n294 = local write "RFID_Error"(w620) -> ()
                n295 = Path To String(path=w606) -> (string=w614:string)
                n296 = To Single Precision Float(number=w633) -> (single precision float=w636:sgl[])
                n297 = xnode "Read/Write Control"("FPGA VI Reference In"=w629, "error in"=w628, "Stop"=TRUE ("stop")) -> ("FPGA VI Reference Out"=w610:refnum<k20>, "error out"=w609:errorcluster)
                n298 = Build Array (concatenate)(w614, w615) -> (w583:string[])
                n299 = local read "TAGS leidos"() -> (w601:path)
                n300 = Write to Binary File(file (use dialog)=w608, data=w636, error in=w632, 5:FALSE ("prepend array or string size? (T)"), 9:T7."little-endian" ("byte order (0:big-endian, network order)")) -> (error out=w605:errorcluster)  [unwired: 3 out]
                n301 = local read "Obstruido?"() -> (w624:bool)
                n302 = for {
                  shift-right: [w665] -> w617
                  shift-left: w605 -> [w664]
                  tunnel: w600 -> [w663] mode=indexing
                  n303 = Close File(refnum=w663, error in=w664) -> (error out=w665:errorcluster)  [unwired: 1 out]
                }
                n304 = call-poly <vilib>:"Write Delimited Spreadsheet.vi"("file path (dialog if empty)"=w601, "1D data"=w583, "append to file? (F)"=FALSE ("transpose? (no:F)"), "transpose? (F)"=TRUE ("append to file? (new file:F)"), "delimiter (\\t)"=";" ("delimiter (\\t)")) -> ()  [unwired: 9 in, 2 out]
                n305 = xnode "Invoke Method"("FPGA VI Reference In"=w610, "error in"=w609) -> ("FPGA VI Reference Out"=w619:refnum<k20>, "error out"=w618:errorcluster)
                n306 = Select(t="Escape", s=w624, f="Procesado") -> (s? t:f=w630:string)
              }
            }
            n307 = call <vilib>:"Watchdog Clear.vi"("error in (no error)"=w373, "watchdogID in"=w374) -> ("error out"=w360:errorcluster)  [unwired: 5 out]
            n308 = Merge Errors(w372, w360) -> (w371:errorcluster)
            n309 = Unbundle By Name(w376) -> ("status"=w358:bool)
            n310 = Unbundle By Name(w372) -> ("status"=w359:bool)
            n311 = Compound Arithmetic op=OR(w358, w359) -> (w356:bool)
            n312 = Select(t="TEST", s=w356, f=w357) -> (s? t:f=w354:string)
          }
          frame "Procesado" {
            n313 = local read "WDOG DISABLE"() -> (w670:bool)
            n314 = local read "WDOG RESET"() -> (w671:bool)
            n315 = call <vilib>:"Watchdog Configure.vi"("RESET"=w671, "error in (no error)"=w692, "expiration actions"="expiration actions", "timeout (1 sec)"=300.0, "DISABLE WDOG"=w670) -> ("error out"=w690:errorcluster, "watchdogID"=w691:u64)  [unwired: 1 in, 2 out]
            n316 = flat-sequence {
              tunnel: w691 -> [w702]
              tunnel: w690 -> [w701]
              tunnel: [w705] -> w674
              tunnel: [w695] -> w673
              tunnel: [w700] -> w672
              tunnel: [w874] -> w688
              tunnel: [w875] -> w689
              tunnel: [w876] -> w685
              tunnel: w674 -> [w876]
              tunnel: w673 -> [w875]
              tunnel: w672 -> [w874]
              frame #0 {
                n317 = flat-sequence {
                  tunnel: [w710] -> w704
                  tunnel: [w726] -> w703
                  tunnel: w702 -> [w749]
                  tunnel: w701 -> [w748]
                  tunnel: [w747] -> w695
                  tunnel: [w746] -> w700
                  tunnel: [w729] -> w699
                  tunnel: [w708] -> w698
                  tunnel: [w728] -> w697
                  tunnel: [w709] -> w696
                  frame #0 {
                    w713 = 3 ("length")
                    # "Estos indicadores sirven para controlar que no se sature la memoria"
                    # "Distancia de\nla unidad"
                    n318 = local read "Nombre de archivo"() -> (w739:path[])
                    n319 = local read "Puntos medios de las ventanas"() -> (w727:dbl[][])
                    n320 = local read "Series del convoy"() -> (w711:string[])
                    n321 = local read "Nº Ejes"() -> (w712:i32[])
                    "Nº Ejes" <- w712
                    n322 = Array Size(array=w739) -> (size(s)=w736:i32)
                    n323 = Add Array Elements(numeric array=w712) -> (sum=w717:i32)
                    "Ejes_convoy" <- w717
                    n324 = Subtract(x=w736, y=1 ("length")) -> (x-y=w738:i32)
                    n325 = Delete From Array(array=w739, index=w738) -> (deleted portion=w735:path, array with subset deleted=w728:path[])  [unwired: 1 in]
                    n326 = local read "Series_flota"() -> (w725:string[])
                    n327 = call <vilib>:"Watchdog Whack.vi"("error in (no error)"=w748, "reset watchdog after expire? (F)"=TRUE, "watchdogID in"=w749) -> ("error out"=w747:errorcluster, "watchdogID out"=w746:u64)  [unwired: 3 out]
                    n328 = Read from Binary File(5:sgl 0.0, 9:T7."little-endian" ("byte order (0:big-endian, network order)"), 10:-1 ("count (1)"), 11:w735) -> (0:w733:errorcluster, 2:w722:sgl[], 3:w734:refnum<file>)  [unwired: 1 in, 2 out]
                    n329 = call "Distancias_ejes_convoy.vi"("Series_flota1"=w711, "Ejes_UT"=w712, "Puntos medios de las ventanas"=w727, "Series_flota"=w725) -> ("Distancias_entre_ejes_convoy"=w726:dbl[])  [unwired: 1 in]
                    n330 = Array Size(array=w722) -> (size(s)=w724:i32)
                    n331 = Subtract(x=w724, y=w713) -> (x-y=w723:i32)
                    n332 = Close File(refnum=w734, error in=w733) -> (error out=w729:errorcluster)  [unwired: 1 out]
                    n333 = Delete From Array(array=w722, length=w713, index=w723) -> (array with subset deleted=w707:sgl[])  [unwired: 1 out]
                    n334 = call "Puntos medio de pulso.vi"("DI Inductivo"=w707) -> ("Puntos"=w710:sgl[], "Número de ejes"=w721:i32)  [unwired: 1 in]
                    "Número de ejes detectados" <- w721
                    n335 = Decrement(x=w721) -> (x-1=w743:i32)
                    n336 = local read "Plataformas?"() -> (w720:bool)
                    n337 = local read "it-LR6"() -> (w716:i32)
                    n338 = local read "it-read-LR6"() -> (w715:i32[])
                    n339 = local read "TAGs LR6"() -> (w714:string[])
                    n340 = local read "TAGs"() -> (w718:string[])
                    n341 = local read "Tiempo de paso (s)"() -> (w742:dbl)
                    n342 = call "Comprobación Señal digital (SubVI).vi"("Inductivo"=w707) -> ("Señal digital?"=w706:bool)
                    "WHEEL_SENSOR" <- w706
                    n343 = call "TAGs_AURAwheel.vi"("Nº Ejes"=w712, "TAGs"=w718, "Ejes_convoy"=w717, "it-LR6"=w716, "TAGs LR6"=w714, "it-read-LR6"=w715, "Plataformas?"=w720) -> ("TAGS_AURA"=→"TAGs_AURAwheel":string[][])  [unwired: 1 in]
                    n344 = call "Calculo_Velocidad.vi"("Tiempo de paso (s)"=w742, "Ejes"=w743, "Puntos iniciales de las ventanas"=w726) -> ("V (m/s)"=→"V (m/s)":dbl, "Longitud de la unidad"=→"Longitud de la unidad":dbl)
                    n345 = Equal?(x=w717, y=w721) -> (x = y?=w709:bool)
                    n346 = Get Volume Info(11:path "c:/" ("path")) -> (1:→"Disco Duro Disponible (bytes)":i64)  [unwired: 1 in, 5 out]
                    n347 = And(x=w709, y=w706) -> (x .and. y?=w708:bool)
                  }
                }
                n348 = case shown="True" w698 {
                  tunnel: w699 -> [w753 w787]
                  tunnel: [w753 w786] -> w705
                  tunnel: w704 -> [_ w791]
                  tunnel: w703 -> [_ w789]
                  tunnel: w697 -> [_ w790]
                  tunnel: w696 -> [w751 _]
                  frame False {
                    n349 = local read "Nombre de archivo"() -> (w752:path[])
                    n350 = for {
                      tunnel: w752 -> [w755] mode=indexing
                      tunnel: w751 -> [w754]
                      n351 = flat-sequence {
                        tunnel: w755 -> [w765]
                        tunnel: [w765] -> w758
                        tunnel: [w764] -> w757
                        tunnel: w754 -> [w761]
                        tunnel: w758 -> [w771]
                        tunnel: [w770] -> w756
                        tunnel: w757 -> [w770]
                        tunnel: w756 -> [w775]
                        frame #0 {
                          w764 = path "c:/Est_Adq.csv" ("file path (use dialog)")
                          n352 = Path To String(path=w765) -> (string=w766:string)
                          n353 = Select(t="Nº Ejes detectados WS diferente a Nº Ejes TAGs" ("delimiter (\\t)"), s=w761, f="La señal del inductivo no es digital" ("delimiter (\\t)")) -> (s? t:f=w760:string)
                          n354 = Build Array(w766, w760) -> (w759:string[])
                          n355 = call-poly <vilib>:"Write Delimited Spreadsheet.vi"("file path (dialog if empty)"=w764, "1D data"=w759, "append to file? (F)"=FALSE ("transpose? (no:F)"), "transpose? (F)"=TRUE ("append to file? (new file:F)"), "delimiter (\\t)"=";" ("delimiter (\\t)")) -> ()  [unwired: 9 in, 2 out]
                        }
                        frame #1 {
                          n356 = disable-structure shown="Disabled" {
                            disable-tunnel: w771 -> [w773 _]
                            frame Disabled {
                              n357 = local read "Digital?"() -> (w772:bool)
                              n358 = case shown="True" w772 {
                                tunnel: w773 -> [_ w774]
                                frame False {
                                }
                                frame True {
                                n359 = Delete(path (use dialog)=w774) -> ()  [unwired: 1 in, 6 out]
                                }
                              }
                            }
                            frame Enabled {
                            }
                          }
                        }
                        frame #2 {
                          n360 = File/Directory Info(path=w775) -> (size=w778:i64)  [unwired: 1 in, 6 out]
                          n361 = Greater?(x=w778, y=i64 1000000) -> (0:w776:bool)
                          n362 = case shown="True" w776 {
                            tunnel: w775 -> [_ w779]
                            frame False {
                            }
                            frame True {
                              n363 = Delete(path (use dialog)=w779) -> ()  [unwired: 4 in, 3 out]
                            }
                          }
                        }
                      }
                    }
                  }
                  frame True {
                    n364 = flat-sequence {
                      tunnel: w791 -> [w860]
                      tunnel: w790 -> [w856]
                      tunnel: w789 -> [w861]
                      tunnel: [w854] -> w784
                      tunnel: [w863] -> w788
                      tunnel: w784 -> [w863]
                      frame #0 {
                        # "Entrada:\n- dt RMS\n- Paths\n- Param_acelerometros (sensivity)\n- Parm_filtro\n- Puntos ventana\n- error\n- Frecuencia\n- Velocidad ejes\n- Punto medio paso rueda (p)"
                        # "SALIDA \n\nMáximos por rueda inductivo"
                        # "ENTRADA \nNúmero de ejes\nDistancia de acelerómetros\nDistancias del centro de las ruedas\nPuntos medios de las ruedas (INDUCTIVO)\nFrecuencia\ndt RMS\nDistancias generales\nAceleraciones"
                        # "8 acelerómetros"
                        # "Velocidad"
                        n365 = local read "Frecuencia de muestreo (Hz)"() -> (w859:dbl)
                        n366 = local read "Distancia de acelerómetros"() -> (w862:dbl[])
                        n367 = local read "Parámetros acelerómetros"() -> (w852:dbl[])
                        n368 = local read "dt RMS"() -> (w858:dbl)
                        n369 = local read "Número de ejes detectados"() -> (w853:i32)
                        n370 = local read "Distancias generales"() -> (w857:dbl[])
                        n371 = call "Procesado_aRMS_Zar.vi"("Número de ejes"=w853, "Distancias generales (m)"=w857, "array"=w856, "Parámetros acelerómetros 2"=w852, "Distancia de acelerómetros"=w862, "Frecuencia de muestreo"=w859, "dt RMS 2"=w858, "Distancias centrales de las ruedas\n               configuración (m)"=w861, "Puntos"=w860) -> ("Max RMS Ruedas"=w855:dbl[][])
                        n372 = Transpose 2D Array(2D array=w855) -> (transposed array=w854:dbl[][])
                        "Max RMS Ruedas" <- w854
                      }
                      frame #1 {
                      }
                    }
                    n373 = local read "TAGs_AURAwheel"() -> (w783:string[][])
                    n374 = local read "Use Aura?"() -> (w782:bool)
                    n375 = local read "Nº Ejes"() -> (w785:i32[])
                    n376 = for {
                      tunnel: w782 -> [w798]
                      tunnel: [w797] -> _ mode=indexing
                      shift-right: [w794] -> _
                      shift-left: w788 -> [w799]
                      tunnel: w783 -> [w796] mode=indexing
                      tunnel: w785 -> [w795] mode=indexing
                      tunnel: [w793] -> w781 mode=indexing
                      tunnel: [w792] -> w780 mode=indexing
                      n377 = case shown="True" w798 {
                        tunnel: w799 -> [w801 w819]
                        tunnel: [w800 w805] -> w797
                        tunnel: w796 -> [_ w812]
                        tunnel: w795 -> [_ w817]
                        tunnel: [w801 w815] -> w794
                        tunnel: [w800 w805] -> w793
                        tunnel: [w800 w802] -> w792
                        frame False {
                          w800 = errorcluster {"status"=FALSE, "code"=0, "source"=""} ("error out")
                        }
                        frame True {
                          w826 = cluster{"status":string} {"status"=""}
                          # "Guardar parámetros\nmedición si falla\ncomunicación"
                          n378 = Delete From Array(array=w819, length=w817, index (row)=0) -> (deleted portion=w818:dbl[][], array with subset deleted=w815:dbl[][])  [unwired: 1 in]
                          n379 = Get Date/Time In Seconds() -> (seconds since 1Jan1904=w847:timestamp)
                          n380 = Format Date/Time String(time format string (%c)="%H:%M:%S%3u", seconds (now)=w847) -> (date/time string=w845:string)  [unwired: 1 in]
                          n381 = Get Date/Time In Seconds() -> (seconds since 1Jan1904=w822:timestamp)
                          n382 = Scan From String(format string="%d:%d:%f", input string=w845) -> (output 1=w842:i32, output 2=w841:i32, output 3=w839:dbl)  [unwired: 5 in, 3 out]
                          n383 = local read "Parametros AuraWheel"() -> (w851:string[])
                          n384 = call "Time_to_ms.vi"("seconds since 1Jan1904"=w822) -> ("Numeric"=w804:dbl)  [unwired: 1 in]
                          n385 = Multiply(x=w839, y=1000.0) -> (x*y=w835:dbl)
                          n386 = Multiply(x=w841, y=60000) -> (x*y=w836:i32)
                          n387 = Multiply(x=3600000, y=w842) -> (x*y=w837:i32)
                          n388 = Compound Arithmetic op=ADD(w837, w836, w835) -> (w834:dbl)
                          n389 = local read "Temperatura (ºC)"() -> (w811:dbl)
                          n390 = To Unsigned Long Integer(number=w834) -> (unsigned 32bit integer=w833:u32)
                          n391 = local read "V (m/s)"() -> (w814:dbl)
                          n392 = Number To Decimal String(number=w833) -> (decimal integer string=w832:string)  [unwired: 1 in]
                          n393 = Index Array(array=w851) -> (element #1=w848:string, element #2=w820:string, element #3=w821:string)  [unwired: 3 in]
                          n394 = Multiply(x=w814, y=3.6) -> (x*y=w809:dbl)
                          n395 = call "aw_WRDCluster_8acel.vi"("Array TAGs"=w812, "Max RMS Ruedas"=w818, "TimeStamp"=w804, "p_sp"=w809, "p_tp"=w811) -> ("JSON cluster"=w810:T9)  [unwired: 1 in]
                          n396 = To Variant(anything=w810) -> (Variant=w831:variant)
                          n397 = call "gjson_Create.vi"("JSON Object in"=w831) -> ("error out"=w829:errorcluster, "JSON String Out"=w830:string)  [unwired: 9 in]
                          n398 = local read "Max RMS Ruedas"() -> (w806:dbl[][])
                          n399 = local read "Temperatura (ºC)"() -> (w808:dbl)
                          n400 = To Variant(anything=w826) -> (Variant=w825:variant)
                          n401 = call "aw_SendData.vi"("pwd"=w848, "x-nem-datetime"=w832, "User"=w820, "error in"=w829, "JSON Object"=w830, "URL"=w821) -> ("error out"=w827:errorcluster, "Response JSON"=w828:string, "Response headers"=→"Response headers":string)  [unwired: 3 in]
                          n402 = local read "V (m/s)"() -> (w807:dbl)
                          n403 = local read "TAGs"() -> (w803:string[])
                          n404 = call "gjson_Parse.vi"("error in"=w827, "JSON String In"=w828, "JSON Cluster"=w825) -> ("error out"=w823:errorcluster, "JSON Cluster Out"=w824:variant)  [unwired: 7 in]
                          n405 = Variant To Data(error in=w823, type=w826, Variant=w824) -> (data=→"data":cluster{"status":string}, error out=w805:errorcluster)
                          "error AURA" <- w805
                          n406 = call "ENVIO_DATOS_AURAWHEEL.vi"("timestamp"=w804, "Array TAGs 2"=w803, "error AURA"=w805, "Max RMS Ruedas"=w806, "p_sp 2"=w807, "p_tp 2"=w808) -> ("error out"=w802:errorcluster)  [unwired: 5 in]
                        }
                      }
                    }
                    n407 = Merge Errors(w781, w780, w787) -> (w786:errorcluster)
                  }
                }
              }
              frame #1 {
                n408 = local read "MB MIN MEMORIA LIBRE"() -> (w865:dbl)
                n409 = local read "MB LIBRE OK"() -> (w864:dbl)
                n410 = local read "Nombre de archivo"() -> (w866:path[])
                n411 = local read "TAGS leidos"() -> (w870:path)
                n412 = File/Directory Info(path=w870) -> (size=w873:i64)  [unwired: 1 in, 6 out]
                n413 = local read "Path TEST"() -> (w869:path)
                n414 = disable-structure shown="Disabled" {
                  frame Disabled {
                    n415 = call "Retrieve_memory_4Gb.vi"() -> ()  [unwired: 12 in]
                  }
                  frame Enabled {
                  }
                }
                n416 = Greater?(x=w873, y=i64 1000000) -> (0:w871:bool)
                n417 = call "Comprimir_a_1_archivo.vi"("Acel_paths"=w866) -> ("path_Pasada"=→"Path Pasada":path)
                n418 = case shown="True" w871 {
                  tunnel: w870 -> [_ w877]
                  frame False {
                  }
                  frame True {
                    n419 = Delete(path (use dialog)=w877) -> ()  [unwired: 4 in, 3 out]
                  }
                }
                n420 = call "Borrar_carpeta.vi"("Nº Archivos Max"=i64 250 ("y"), "Path Carpeta"=w869) -> ()  [unwired: 1 in]
                n421 = call "BORRADO_MEJORADO.vi"("MB LIBRE OK"=w864, "MB Minimo de Memoria libre"=w865) -> ()  [unwired: 10 in]
              }
            }
            n422 = local read "RFID_Error"() -> (w675:errorcluster)
            n423 = call <vilib>:"Watchdog Clear.vi"("error in (no error)"=w689, "watchdogID in"=w688) -> ("error out"=w687:errorcluster)  [unwired: 5 out]
            n424 = Merge Errors(w685, w687) -> (w676:errorcluster)
            n425 = Merge Errors(w669, w675) -> (w686:errorcluster)
            n426 = Unbundle By Name(w686) -> ("status"=w680:bool)
            n427 = Select(t="Descarga datos", s=FALSE, f="Espera") -> (s? t:f=w682:string)
            n428 = Select(t="TEST", s=w680, f=w682) -> (s? t:f=w679:string)
          }
          frame "TEST" {
            # "Enviar estado de salud\nde WRD a AURA wheel"
            n429 = local read "WHEEL_SENSOR"() -> (w889:bool)
            n430 = local read "Max RMS Ruedas"() -> (w888:dbl[][])
            n431 = local read "Parametros AuraWheel"() -> (w878:string[])
            n432 = local read "T fuera rango"() -> (w890:bool)
            n433 = local read "RFID_Error"() -> (w892:errorcluster)
            n434 = local read "Fallo fotocelula"() -> (w891:bool)
            n435 = local read "RFID_LR6_Error"() -> (w893:errorcluster)
            n436 = call "pRUEBA_JSON.vi"("TEMPERATURA"=w890, "Parametros AuraWheel"=w878, "all rows"=w888, "WHEEL_SENSOR"=w889, "LIMITE MAX"="LIMITE MAX", "LIMITE MIN"="LIMITE MIN", "RFID_Error"=w892, "FOTOCELULA"=w891, "RFID_LR6_Error"=w893, "ESCRITURA ERROR"=w895, "FPGA ERROR"=w894) -> ("JSON String Out"=→"JSON String Out":string, "Response headers"=w880:string, "error AURA"=w879:errorcluster)  [unwired: 6 in]
            n437 = local write "error AURA"(w879) -> ()
            n438 = local write "Response headers"(w880) -> ()
            n439 = local read "WDOG DISABLE"() -> (w885:bool)
            n440 = local read "expiration actions"() -> (w896:T1)
            n441 = local read "WDOG RESET"() -> (w884:bool)
            n442 = call <vilib>:"Watchdog Configure.vi"("RESET"=w884, "expiration actions"=w896, "timeout (1 sec)"=100.0, "DISABLE WDOG"=w885) -> ("error out"=w899:errorcluster, "watchdogID"=w900:u64)  [unwired: 2 in, 2 out]
            n443 = flat-sequence {
              tunnel: [w910] -> w905
              tunnel: w895 -> [w930]
              tunnel: w894 -> [w929]
              tunnel: [w928] -> w883
              tunnel: w900 -> [w919]
              tunnel: w899 -> [w918]
              tunnel: [w917] -> w898
              tunnel: [w916] -> w897
              tunnel: [w906] -> w903
              frame #0 {
                n444 = call <vilib>:"Watchdog Whack.vi"("error in (no error)"=w918, "reset watchdog after expire? (F)"=TRUE, "watchdogID in"=w919) -> ("error out"=w916:errorcluster, "watchdogID out"=w917:u64)  [unwired: 3 out]
                n445 = Get Date/Time In Seconds() -> (seconds since 1Jan1904=w922:timestamp)
                n446 = local read "Ultimo TEST"() -> (w923:timestamp)
                n447 = To Double Precision Float(number=w922) -> (double precision float=w924:dbl)
                n448 = Subtract(x=w924, y=3600.0) -> (x-y=w926:dbl)
                n449 = To Time Stamp(1:w926) -> (0:w927:timestamp)
                n450 = In Range and Coerce(upper limit=w922, x=w923, lower limit=w927) -> (In Range?=w921:bool)  [unwired: 1 out]
                n451 = case shown="False" w921 {
                  tunnel: w930 -> [w932 _]
                  tunnel: w929 -> [w931 w966]
                  tunnel: [w946 errorcluster {"status"=FALSE, "code"=0, "source"=""} ("error out")] -> w928
                  tunnel: [w931 w966] -> w906
                  frame False {
                    n452 = local read "Obstruido?"() -> (w938:bool)
                    n453 = local read "Aviso no detección"() -> (w944:string)
                    n454 = case shown="True" w938 {
                      selector: w938 -> [_ w962]
                      tunnel: ["\r" w963] -> w933
                      frame False {
                      }
                      frame True {
                        n455 = call "ErrorObstruccion.vi"("Buffer Overflow"=w962) -> ("error out"=w965:errorcluster)
                        n456 = call "Error.vi"("Error con..."="Warning:", "error comunicacion 2"=w965) -> ("String"=w963:string)
                      }
                    }
                    n457 = local read "Aviso temperatura"() -> (w943:string)
                    n458 = local read "RFID_LR6_Error"() -> (w936:errorcluster)
                    n459 = local read "RFID_Error"() -> (w940:errorcluster)
                    n460 = local read "DC OK"() -> (w942:string)
                    n461 = local read "Fallo sensores"() -> (w937:string)
                    n462 = call "Cabecera.vi"() -> ("String"=w959:string)
                    n463 = call "Adquisicion.vi"("Aviso no detección"=w944) -> ("String"=w958:string)
                    n464 = call "Temperatura.vi"("Aviso temperatura"=w943) -> ("String"=w957:string)
                    n465 = call "Fuente.vi"("DC OK"=w942) -> ("String"=w956:string)
                    n466 = call "FPGA.vi"("error out"=w931) -> ("String"=w955:string)
                    n467 = call "Escritura.vi"("error out"=w932) -> ("String"=w954:string)
                    n468 = call "Error.vi"("Error con..."="Error con el lector RFID LR6-HD", "error comunicacion 2"=w936) -> ("String"=w934:string)
                    n469 = call "Error.vi"("Error con..."="Error con el lector RFID NEM", "error comunicacion 2"=w940) -> ("String"=w939:string)
                    n470 = Concatenate Strings(w959, w958, w957, w956, w955, w954, w937, w939, w934, w933) -> (w960:string)
                    n471 = call "STRINGhorafechA(SubVI).vi"() -> ("STRINGhora_fecha"=w953:string)
                    n472 = Concatenate Strings(w953, ".txt" ("string")) -> (w949:string)
                    n473 = Build Array("c", "TEST" ("element"), w949) -> (w951:string[])
                    n474 = Get Date/Time In Seconds() -> (seconds since 1Jan1904=→"Ultimo TEST":timestamp)
                    n475 = Array of Strings to Path(0:w951) -> (2:w947:path)  [unwired: 1 out]
                    n476 = Write to Text File(file (use dialog)=w947, text=w960) -> (error out=w946:errorcluster)  [unwired: 1 in, 3 out]
                  }
                  frame True {
                  }
                }
                n477 = local read "Fallo fotocelula"() -> (w909:bool)
                n478 = local read "T fuera rango"() -> (w915:bool)
                n479 = Unbundle By Name(w906) -> ("status"=w907:bool)
                n480 = Compound Arithmetic op=OR(w907, w909) -> (w908:bool)
                n481 = local write "Reset del controlador"(w908) -> ()
                n482 = Select(t="Escape", s=w915, f="Espera") -> (s? t:f=w912:string)
                n483 = Select(t="Configuracion", s=w908, f=w912) -> (s? t:f=w910:string)
              }
            }
            n484 = call <vilib>:"Watchdog Clear.vi"("error in (no error)"=w897, "watchdogID in"=w898) -> ("error out"=w882:errorcluster)  [unwired: 5 out]
            n485 = Merge Errors(w883, w882) -> (w881:errorcluster)
          }
          frame "Escape" {
            n486 = while {
              shift-right: [w987] -> w972
              shift-left: w971 -> [w986]
              shift-right: [w985] -> w969
              shift-left: w968 -> [w984]
              stop <- w974 stop-if-true
              # "Espera hasta que el detector de\npresencia se desactive"
              n487 = Wait (ms)(milliseconds to wait=u32 3000) -> ()  [unwired: 1 out]
              n488 = xnode "Read/Write Control"("FPGA VI Reference In"=w986, "error in"=w984) -> ("FPGA VI Reference Out"=w987:refnum<k20>, "error out"=w985:errorcluster, "Detector de presencia"=w982:bool, "Chassis Temperature"=w977:i16)
              n489 = Divide(x=w977, y=4.0) -> (x/y=w978:dbl)
              n490 = In Range and Coerce(upper limit=55.0, x=w978, lower limit=0.0) -> (In Range?=w975:bool)  [unwired: 1 out]
              n491 = Not(x=w982) -> (.not. x?=w976:bool)
              n492 = And(x=w976, y=w975) -> (x .and. y?=w974:bool)
            }
          }
          frame "SUBIDA_FALLOS_AW" {
            n493 = flat-sequence {
              tunnel: [w1023] -> w996
              tunnel: [w1022] -> w995
              tunnel: w998 -> [w1017]
              tunnel: w1005 -> [w1022]
              tunnel: w1007 -> [w1023]
              tunnel: [w1015] -> w993
              tunnel: [w1009] -> w989
              tunnel: [w1086] -> w1006
              tunnel: [w1087] -> w994
              tunnel: w996 -> [w1087]
              tunnel: w995 -> [w1086]
              tunnel: w993 -> [w1085]
              tunnel: [w1085] -> w992
              tunnel: w989 -> [w1084]
              tunnel: [w1084] -> w988
              frame #0 {
                n494 = local read "expiration actions"() -> (w1013:T1)
                n495 = local read "WDOG DISABLE"() -> (w1011:bool)
                n496 = local read "WDOG RESET"() -> (w1012:bool)
                n497 = call <vilib>:"Watchdog Configure.vi"("RESET"=w1012, "error in (no error)"=w1017, "expiration actions"=w1013, "timeout (1 sec)"=200.0, "DISABLE WDOG"=w1011) -> ("error out"=w1016:errorcluster, "watchdogID"=w1010:u64)  [unwired: 1 in, 2 out]
                n498 = call-poly <vilib>:"Read Delimited Spreadsheet.vi"("file path (dialog if empty)"=path "C:/MEDIDAS_PENDIENTES/AURA_WHEEL.csv", "format (%s)"="%s", "delimiter (\\t)"=";" ("delimiter (\\t)")) -> ("all rows"=w1018:string[][])  [unwired: 7 in, 5 out]
                "all rows" <- w1018
                n499 = while {
                  shift-right: [w1030] -> _
                  shift-left: w1018 -> [w1083]
                  tunnel: w1016 -> [w1027]
                  tunnel: [w1026] -> w1015
                  tunnel: w1010 -> [w1025]
                  tunnel: [w1024] -> w1009
                  stop <- w1082 stop-if-true
                  w1053 = cluster{"status":string} {"status"=""}
                  n500 = call "VARIABLES_FALLOS.vi"("all rows"=w1083) -> ("MAX RMS RUEDAS"=w1071:dbl[][], "all rows 4"=w1030:string[][], "TAGS"=w1073:string[][], "TIMESTAMP"=w1074:dbl[], "VELOCIDAD"=w1072:dbl[], "TEMPER"=w1075:dbl[])  [unwired: 4 in, 1 out]
                  n501 = call "ARRAY VARIABLES.vi"("TIMESTAMP"=w1074, "VELOCIDAD"=w1072, "TAGS"=w1073, "TEMPER"=w1075) -> ("ARRAY TAGS"=w1079:string[], "ARRAY TIMESTAMP"=w1078:dbl, "ARRAY VELOCIDAD"=w1077:dbl, "TEMPERATURA"=w1076:dbl)  [unwired: 4 in]
                  n502 = call <vilib>:"Watchdog Whack.vi"("error in (no error)"=w1027, "reset watchdog after expire? (F)"=TRUE, "watchdogID in"=w1025) -> ("error out"=w1026:errorcluster, "watchdogID out"=w1024:u64)  [unwired: 3 out]
                  n503 = call "aw_WRDCluster_8acel_FALLOS_SUBIDA.vi"("Array TAGs"=w1079, "Max RMS Ruedas"=w1071, "TimeStamp"=w1078, "p_sp"=w1077, "p_tp"=w1076) -> ("JSON cluster"=w1080:T9)  [unwired: 1 in]
                  n504 = To Variant(anything=w1080) -> (Variant=w1081:variant)
                  n505 = call "gjson_Create.vi"("JSON Object in"=w1081) -> ("error out"=w1034:errorcluster, "JSON String Out"=w1035:string)  [unwired: 9 in]
                  "JSON String Out 2" <- w1035
                  n506 = Get Date/Time In Seconds() -> (seconds since 1Jan1904=w1038:timestamp)
                  n507 = Index Array(array="Parametros AuraWheel 2") -> (element #1=w1059:string, element #2=w1060:string, element #3=w1061:string)  [unwired: 3 in]
                  n508 = Format Date/Time String(time format string (%c)="%H:%M:%S%3u", seconds (now)=w1038) -> (date/time string=w1040:string)  [unwired: 1 in]
                  n509 = Scan From String(format string="%d:%d:%f", input string=w1040) -> (output 1=w1043:i32, output 2=w1044:i32, output 3=w1046:dbl)  [unwired: 5 in, 3 out]
                  n510 = Multiply(x=w1046, y=1000.0) -> (x*y=w1050:dbl)
                  n511 = Multiply(x=w1044, y=60000) -> (x*y=w1049:i32)
                  n512 = Multiply(x=3600000, y=w1043) -> (x*y=w1048:i32)
                  n513 = Compound Arithmetic op=ADD(w1048, w1049, w1050) -> (w1051:dbl)
                  n514 = To Variant(anything=w1053) -> (Variant=w1054:variant)
                  n515 = To Unsigned Long Integer(number=w1051) -> (unsigned 32bit integer=w1052:u32)
                  n516 = Number To Decimal String(number=w1052) -> (decimal integer string=w1062:string)  [unwired: 1 in]
                  n517 = call "aw_SendData.vi"("pwd"=w1059, "x-nem-datetime"=w1062, "User"=w1060, "error in"=w1034, "JSON Object"=w1035, "URL"=w1061) -> ("error out"=w1057:errorcluster, "Response JSON"=w1058:string, "Response headers"=→"Response headers 2":string)  [unwired: 3 in]
                  n518 = call "gjson_Parse.vi"("error in"=w1057, "JSON String In"=w1058, "JSON Cluster"=w1054) -> ("error out"=w1056:errorcluster, "JSON Cluster Out"=w1055:variant)  [unwired: 7 in]
                  n519 = Variant To Data(error in=w1056, type=w1053, Variant=w1055) -> (data=→"data 2":cluster{"status":string}, error out=→"error out":errorcluster)
                  n520 = Array Size(array=w1030) -> (size(s)=w1032:i32[])
                  n521 = Delete From Array(array=w1032) -> (array with subset deleted=w1031:i32[])  [unwired: 2 in, 1 out]
                  n522 = Delete From Array(array=w1031) -> (deleted portion=w1029:i32)  [unwired: 2 in, 1 out]
                  n523 = local read "HORA_FINAL_SUBIDA"() -> (w1067:string)
                  n524 = Get Date/Time In Seconds() -> (seconds since 1Jan1904=w1068:timestamp)
                  n525 = Get Date/Time String(seconds (now)=w1068, want seconds? (F)=TRUE) -> (time string=w1066:string)  [unwired: 1 in, 1 out]
                  n526 = Equal?(x=w1067, y=w1066) -> (x = y?=w1065:bool)
                  n527 = Less?(x=w1029, y=1) -> (x < y?=w1069:bool)
                  n528 = Or(x=w1069, y=w1065) -> (x .or. y?=w1082:bool)
                }
              }
              frame #1 {
              }
            }
            n529 = Unbundle By Name(w994) -> ("status"=w999:bool)
            n530 = Merge Errors(w994, w992) -> (w991:errorcluster)
            n531 = local read "T fuera rango"() -> (w1004:bool)
            n532 = Compound Arithmetic op=OR(w999) -> (w1000:bool)
            n533 = Select(t="Escape", s=w1004, f="Espera") -> (s? t:f=w1002:string)
            n534 = Select(t="Configuracion", s=w1000, f=w1002) -> (s? t:f=w1008:string)
            n535 = call <vilib>:"Watchdog Clear.vi"("error in (no error)"=w991, "watchdogID in"=w988) -> ("error out"=w990:errorcluster)  [unwired: 5 out]
          }
        }
        "Estado" <- w82
        "error manipulacion archivos" <- w84
        n536 = local read "Parar la aplicación"() -> (w81:bool)
      }
      n537 = xnode "Close FPGA VI Reference"("FPGA VI Reference In"=w74, "error in"=w73) -> ("error out"=→"error FPGA":errorcluster)
    }
    frame #3 {
      n538 = local read "RFID_NEM_On"() -> (w1089:bool)
      n539 = local read "RFID_GEN_On"() -> (w1088:bool)
      n540 = case shown="True" w1089 {
        frame False {
        }
        frame True {
          n541 = local read "RFID_ID"() -> (w1092:refnum<k5>)
          n542 = TCP Close Connection(connection ID=w1092) -> (error out=→"RFID_Error":errorcluster)  [unwired: 1 in, 2 out]
        }
      }
      n543 = case shown="True" w1088 {
        frame False {
        }
        frame True {
          n544 = call "LH6HD.vi"("Action"=enum16{"Init", "Start", "Read", "Stop", "Exit"}."Stop") -> ("error out"=→"RFID_LR6_Error":errorcluster)  [unwired: 9 in, 1 out]
        }
      }
    }
  }
